vi "Actor Core.vi"(8 "error in":errorcluster, 11 "Zen Analytics in":refnum<class "Zen Analytics.lvclass">) -> (0 "error out":errorcluster, 3 "Actor out":refnum<class "Actor.lvclass">)   [LabVIEW 2019, in "Zen Analytics.lvlib" / "Zen Analytics.lvclass"]
doc: "(<B>Filename</B>: Actor Framework.lvlib:Actor.lvclass:Actor Core.vi)\n\nReceives messages to the actor, reacts to them, and initiates any error handling that may shut the actor down.\n\nDescendant classes may override this VI to append parallel tasks for the actor to complete while it handles messages. Overrides use the Call Parent Method node."
uses:
  Zen Analytics.lvclass
  <vilib>/ActorFramework/Actor/Actor.lvclass
  <vilib>/ActorFramework/Message Enqueuer/Message Enqueuer.lvclass
  Dependency/Plot Cluster.ctl
  Dependency/GraphReff.ctl
  Dependency/Initialize_Cluster.ctl
  Dependency/JSON Cluster(Int).ctl
  Dependency/Shift Registers Cluster.ctl
  <vilib>/ActorFramework/Stop Msg/Stop Msg.lvclass
  Dependency/AnalyticsDataToSM.ctl
  <userlib>/_OpenG.lib/array/array.llb/Empty Array (Variant)__ogtk.vi
  C:/Program Files/National Instruments/LabVIEW 2019/vi.lib/ActorFramework/Actor/Actor.lvclass
panel:
  out "Terminal Count":u32
  out "Reduced 2D":dbl[][](array[numeric])
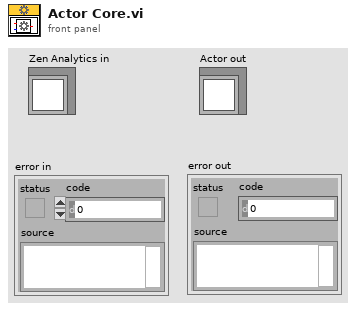
[diagram p1: front panel]
types:
  T1 = cluster{"InitializationParams":cluster{"ColumnNo":i32, "MeasurementData":cluster{"Measurement ID":i32, "Measurement Name":string, "Nominal Values":dbl, "LSL":dbl, "USL":dbl, "LCL":dbl, "UCL":dbl}[]}}
  T2 = enum32{"invalid app kind", "Development System", "Run Time System", "Student Edition", "Embedded LabVIEW", "Evaluation", "Custom"}
  T3 = enum32{"Invalid", "Standard", "Closed", "Hidden", "Minimized", "Maximized"}
  T4 = typedef "Zen Analytics.lvlib/Zen Analytics.lvclass/AnalyticsDataToSM.ctl" = cluster{"Actor Info":cluster{"Analytics Enqueuer":refnum<class "Message Enqueuer.lvclass">, "This VI":refnum<vi>, "Module name":string}, "Statistical Info":string[][], "Graph Refference's":T5, "ErrorMessage":string}
  T5 = typedef "Zen Analytics.lvlib/Zen Analytics.lvclass/GraphReff.ctl" = cluster{"HistgramGraph-reff":refnum<vi>[], "BarGraph-reff":refnum<vi>[], "PieGraph-reff":refnum<vi>[], "Lable-reff":refnum<vi>[], "TrendGraph-reff":refnum<vi>[], "CpCpkTable":refnum<vi>}
  T6 = cluster{"InitializationParams":cluster{"CurrentPartNumber":string, "Re-Initialize?":bool, "MeasurementData":cluster{"Measurement ID":i32, "Measurement Name":string, "Nominal Values":dbl, "LSL":dbl, "USL":dbl, "LCL":dbl, "UCL":dbl}[]}}
  T7 = cluster{"SumOfSquareOfData":dbl, "SumOfMeasurementData":dbl, "N ":u32}
  T8 = typedef "Zen Analytics.lvlib/Zen Analytics.lvclass/Shift Registers Cluster.ctl" = cluster{"Initialize 2D Array":dbl[][], "Analytics Button Pressed?":bool, "Analytics Or Back?":bool, "Read Config":bool, "Prev Terminal Count":u32, "Plot:Present Terminal":u32, "Timeout?":bool, "Re-initialized":bool}
  T9 = typedef "Zen Analytics.lvlib/Zen Analytics.lvclass/JSON Cluster(Int).ctl" = cluster{"Rows In 2D Array":i32, "Columns In 2D Array":i32, "Samples To Display":i32, "Update Rate (Time)":i32, "Update Rate (Samples)":i32, "CurrentPartNumber":string, "AnalyticsDataFormat":cluster{"AnalyticsParameters":cluster{"UpdateRateCategories":cluster{"LOW":cluster{"SampleElapsed":dbl, "TimeElapsed":dbl}, "MEDIUM":cluster{"SampleElapsed":dbl, "TimeElapsed":dbl}, "HIGH":cluster{"SampleElapsed":dbl, "TimeElapsed":dbl}}, "AnalyticsForPartsList":cluster{"Name":string, "InitializationValues":cluster{"RowsIn2DArray":dbl, "ColumnsIn2DArray":dbl, "SamplesToDisplay":dbl, "UpdateRate":string}, "PlotParameters":cluster{"Trend":cluster{"TrendPlotID":dbl, "PlotProperties":cluster{"FontName":string, "FontSize":dbl, "FontColor":string, "IsBold":bool, "IsItalic":bool, "PlotColor":string}}[], "Histogram":cluster{"HistogramPlotID":dbl, "PlotProperties":cluster{"FontName":string, "FontSize":dbl, "FontColor":string, "IsBold":bool, "IsItalic":bool, "PlotColor":string}}[], "BarPlot":cluster{"BarPlotID":dbl, "BarValuesID":dbl, "PlotProperties":cluster{"FontName":string, "FontSize":dbl, "IsBold":bool, "IsItalic":bool, "FontColor":string}, "Sectors":string[]}[], "PieChart":cluster{"PieChartID":dbl, "PieChartValueID":dbl, "PlotProperties":cluster{"FontName":string, "FontSize":dbl, "IsBold":bool, "IsItalic":bool, "FontColor":string}, "Sectors":string[]}[]}}[]}}, "MeasurementData":cluster{"Measurement ID":i32, "Measurement Name":string, "Nominal Values":dbl, "LSL":dbl, "USL":dbl, "LCL":dbl, "UCL":dbl}[], "PlotParameters":cluster{"Trend":cluster{"TrendPlotID":dbl, "PlotProperties":cluster{"FontName":string, "FontSize":dbl, "FontColor":string, "IsBold":bool, "IsItalic":bool, "PlotColor":string}}[], "Histogram":cluster{"HistogramPlotID":dbl, "PlotProperties":cluster{"FontName":string, "FontSize":dbl, "FontColor":string, "IsBold":bool, "IsItalic":bool, "PlotColor":string}}[], "BarPlot":cluster{"BarPlotID":dbl, "BarValuesID":dbl, "PlotProperties":cluster{"FontName":string, "FontSize":dbl, "IsBold":bool, "IsItalic":bool, "FontColor":string}, "Sectors":string[]}[], "PieChart":cluster{"PieChartID":dbl, "PieChartValueID":dbl, "PlotProperties":cluster{"FontName":string, "FontSize":dbl, "IsBold":bool, "IsItalic":bool, "FontColor":string}, "Sectors":string[]}[]}}
  T10 = typedef "Zen Analytics.lvlib/Zen Analytics.lvclass/Initialize_Cluster.ctl" = cluster{"Initialization Values ":cluster{"InitializationParams":cluster{"CurrentPartNumber":string, "Re-Initialize?":bool, "MeasurementData":cluster{"Measurement ID":i32, "Measurement Name":string, "Nominal Values":dbl, "LSL":dbl, "USL":dbl, "LCL":dbl, "UCL":dbl}[]}}}
  T11 = typedef "Zen Analytics.lvlib/Zen Analytics.lvclass/Plot Cluster.ctl" = cluster{"Reduced 2D":dbl[][], "Start Index":i32, "No Of New Termnals":i32, "Top/Bottom":bool, "Values Inserted":i32, "Re-Initialised":bool, "Statistical params":string[][], "MeasurementInitializationData":cluster{"Measurement-ID":i32[], "Measurement Names":string[], "NominalValues":dbl[], "LSL":dbl[], "USL":dbl[], "LCL":dbl[], "UCL":dbl[]}, "MeasurementData":cluster{"Measurement ID":i32, "Measurement Name":string, "Nominal Values":dbl, "LSL":dbl, "USL":dbl, "LCL":dbl, "UCL":dbl}[], "ResultData2D":dbl[][], "PlotParameters":cluster{"Trend":cluster{"TrendPlotID":dbl, "PlotProperties":cluster{"FontName":string, "FontSize":dbl, "FontColor":string, "IsBold":bool, "IsItalic":bool, "PlotColor":string}}[], "Histogram":cluster{"HistogramPlotID":dbl, "PlotProperties":cluster{"FontName":string, "FontSize":dbl, "FontColor":string, "IsBold":bool, "IsItalic":bool, "PlotColor":string}}[], "BarPlot":cluster{"BarPlotID":dbl, "BarValuesID":dbl, "PlotProperties":cluster{"FontName":string, "FontSize":dbl, "IsBold":bool, "IsItalic":bool, "FontColor":string}, "Sectors":string[]}[], "PieChart":cluster{"PieChartID":dbl, "PieChartValueID":dbl, "PlotProperties":cluster{"FontName":string, "FontSize":dbl, "IsBold":bool, "IsItalic":bool, "FontColor":string}, "Sectors":string[]}[]}}
  T12 = cluster{"Core":cluster{"Current VI Reference":refnum<vi>, "Close Panel on Exit?":bool}, "clusterForShiftReg":T8, "JSON Cluster":T9, "Initialization Values":T10, "ResultCluster":cluster{"Terminal Count":u32, "isPass":bool, "Terminal Data 1D":dbl[], "Defect":bool[]}, "Pause Data":bool, "Statistical Parameters":string[][], "InitializationValues":dbl[][], "InitializationValue-PieCahrt":cluster{"InitializationDefect":dbl[], "InitializationProduction":dbl[]}, "InitializationValue-Barplot":cluster{"InitializationDefect":dbl[], "InitializationProduction":dbl[]}, "GraphRefference":T5, "Count":i32, "A_Count":i32, "Data & ID's":cluster{"Measurement-ID":i32[], "Measurement Names":string[], "NominalValues":dbl[], "LSL":dbl[], "USL":dbl[], "LCL":dbl[], "UCL":dbl[]}, "IndexOfMeasurement":i32, "Plot Cluster":T11, "InitializationValues_New":dbl[][], "InterActorData":variant, "StatDataIn ":cluster{"SumOfSquareOfData":dbl, "SumOfMeasurementData":dbl, "N ":u32}[], "StatData Old":cluster{"SumOfSquareOfData":dbl, "SumOfMeasurementData":dbl, "N ":u32}[], "oldTerminalCount":i32}
  T13 = cluster{"SumOfSquareOfData":dbl, "SumOfMeasurementData":dbl, "N ":u32}[]
  T14 = cluster{"Measurement-ID":i32[], "Measurement Names":string[], "NominalValues":dbl[], "LSL":dbl[], "USL":dbl[], "LCL":dbl[], "UCL":dbl[]}
  T15 = cluster{"InitializationDefect":dbl[], "InitializationProduction":dbl[]}
  T16 = cluster{"Terminal Count":u32, "isPass":bool, "Terminal Data 1D":dbl[], "Defect":bool[]}
  T17 = cluster{"Current VI Reference":refnum<vi>, "Close Panel on Exit?":bool}
  T18 = cluster{"AnalyticsParameters":cluster{"UpdateRateCategories":cluster{"LOW":cluster{"SampleElapsed":dbl, "TimeElapsed":dbl}, "MEDIUM":cluster{"SampleElapsed":dbl, "TimeElapsed":dbl}, "HIGH":cluster{"SampleElapsed":dbl, "TimeElapsed":dbl}}, "AnalyticsForPartsList":cluster{"Name":string, "InitializationValues":cluster{"RowsIn2DArray":dbl, "ColumnsIn2DArray":dbl, "SamplesToDisplay":dbl, "UpdateRate":string}, "PlotParameters":cluster{"Trend":cluster{"TrendPlotID":dbl, "PlotProperties":cluster{"FontName":string, "FontSize":dbl, "FontColor":string, "IsBold":bool, "IsItalic":bool, "PlotColor":string}}[], "Histogram":cluster{"HistogramPlotID":dbl, "PlotProperties":cluster{"FontName":string, "FontSize":dbl, "FontColor":string, "IsBold":bool, "IsItalic":bool, "PlotColor":string}}[], "BarPlot":cluster{"BarPlotID":dbl, "BarValuesID":dbl, "PlotProperties":cluster{"FontName":string, "FontSize":dbl, "IsBold":bool, "IsItalic":bool, "FontColor":string}, "Sectors":string[]}[], "PieChart":cluster{"PieChartID":dbl, "PieChartValueID":dbl, "PlotProperties":cluster{"FontName":string, "FontSize":dbl, "IsBold":bool, "IsItalic":bool, "FontColor":string}, "Sectors":string[]}[]}}[]}}
  T19 = cluster{"Trend":cluster{"TrendPlotID":dbl, "PlotProperties":cluster{"FontName":string, "FontSize":dbl, "FontColor":string, "IsBold":bool, "IsItalic":bool, "PlotColor":string}}[], "Histogram":cluster{"HistogramPlotID":dbl, "PlotProperties":cluster{"FontName":string, "FontSize":dbl, "FontColor":string, "IsBold":bool, "IsItalic":bool, "PlotColor":string}}[], "BarPlot":cluster{"BarPlotID":dbl, "BarValuesID":dbl, "PlotProperties":cluster{"FontName":string, "FontSize":dbl, "IsBold":bool, "IsItalic":bool, "FontColor":string}, "Sectors":string[]}[], "PieChart":cluster{"PieChartID":dbl, "PieChartValueID":dbl, "PlotProperties":cluster{"FontName":string, "FontSize":dbl, "IsBold":bool, "IsItalic":bool, "FontColor":string}, "Sectors":string[]}[]}
  T20 = cluster{"Measurement ID":i32, "Measurement Name":string, "Nominal Values":dbl, "LSL":dbl, "USL":dbl, "LCL":dbl, "UCL":dbl}[]
  T21 = typedef "Zen Analytics.lvlib/Zen Analytics.lvclass/Json Partno Specific output.ctl" = cluster{"Array Params ":cluster{"RowsIn2DArray":i32, "ColumnsIn2DArray":i32, "SamplesToDisplay":i32, "UpdateRate":string}, "PlotParameters":cluster{"Trend":cluster{"TrendPlotID":dbl, "PlotProperties":cluster{"FontName":string, "FontSize":dbl, "FontColor":string, "IsBold":bool, "IsItalic":bool, "PlotColor":string}}[], "Histogram":cluster{"HistogramPlotID":dbl, "PlotProperties":cluster{"FontName":string, "FontSize":dbl, "FontColor":string, "IsBold":bool, "IsItalic":bool, "PlotColor":string}}[], "BarPlot":cluster{"BarPlotID":dbl, "BarValuesID":dbl, "PlotProperties":cluster{"FontName":string, "FontSize":dbl, "IsBold":bool, "IsItalic":bool, "FontColor":string}, "Sectors":string[]}[], "PieChart":cluster{"PieChartID":dbl, "PieChartValueID":dbl, "PlotProperties":cluster{"FontName":string, "FontSize":dbl, "IsBold":bool, "IsItalic":bool, "FontColor":string}, "Sectors":string[]}[]}}
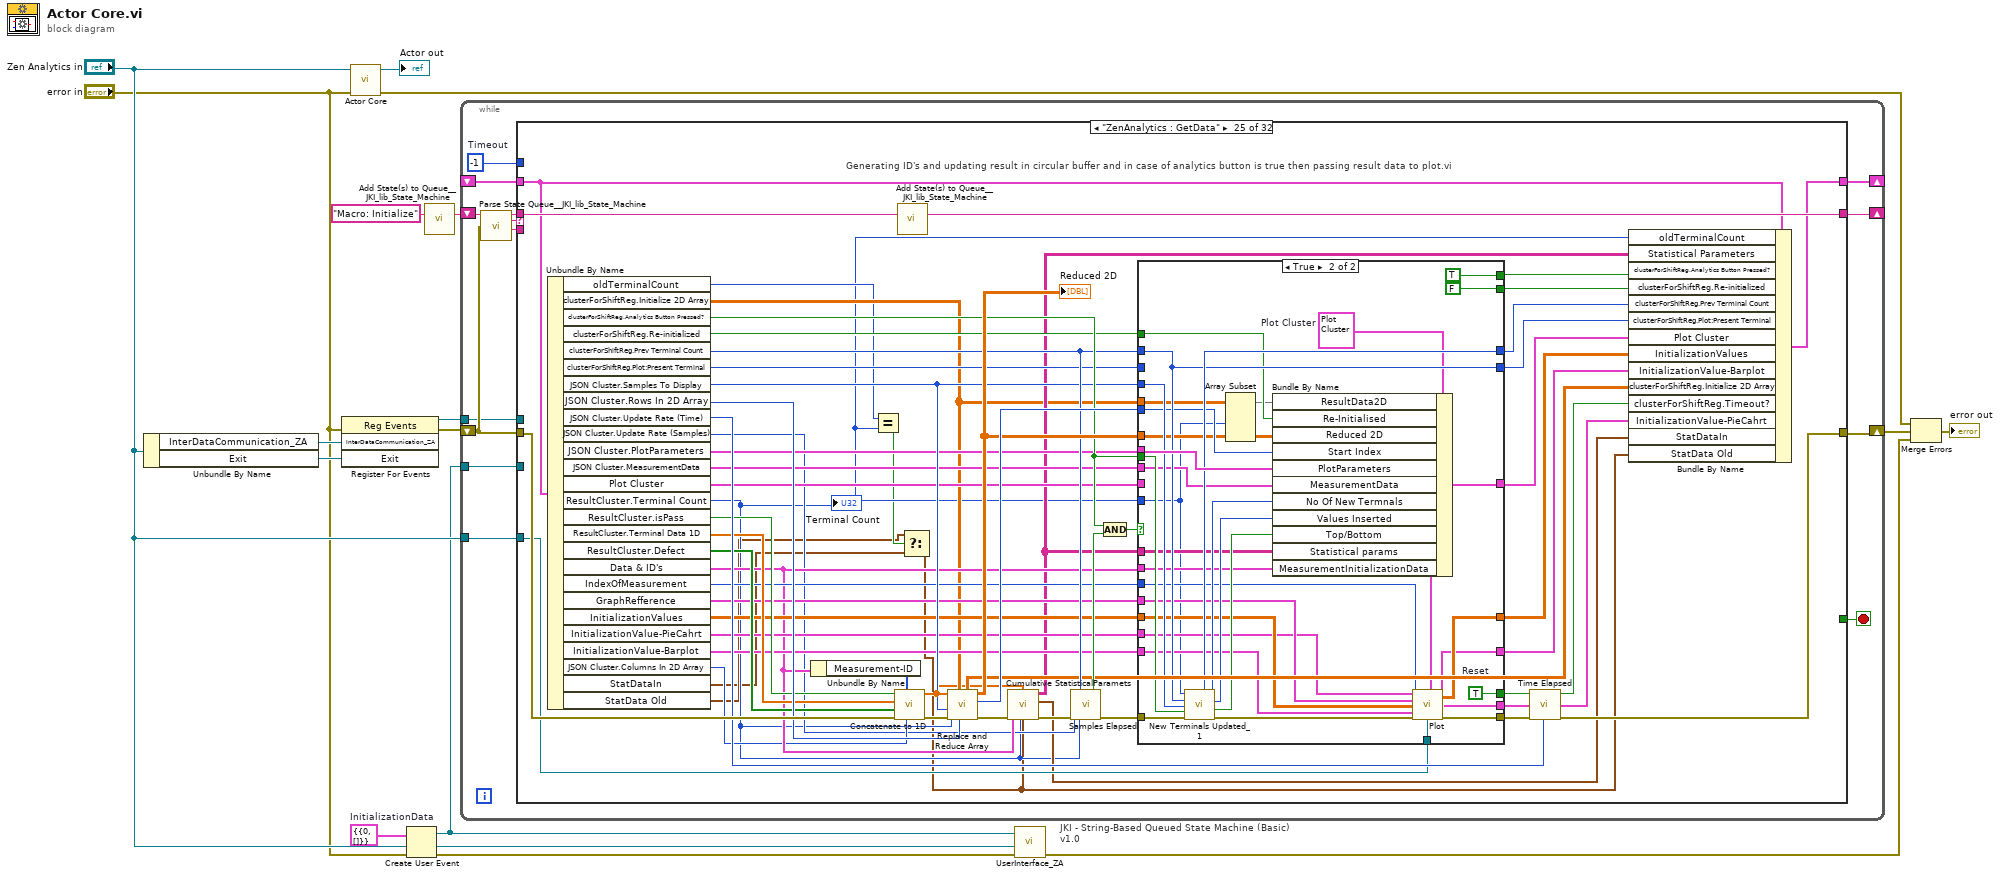
[diagram p0: block diagram]
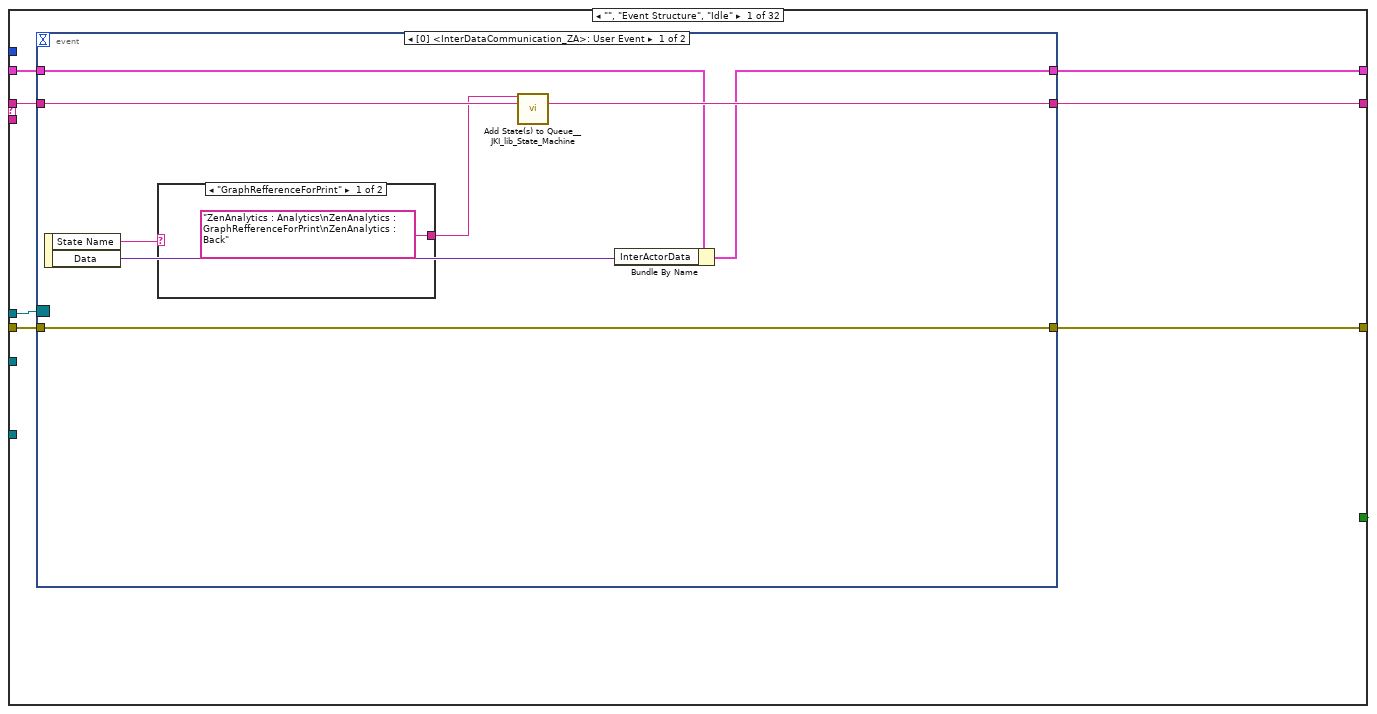
[diagram p2: hidden frame]
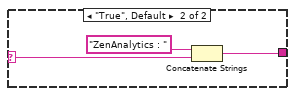
[diagram p3: hidden frame]
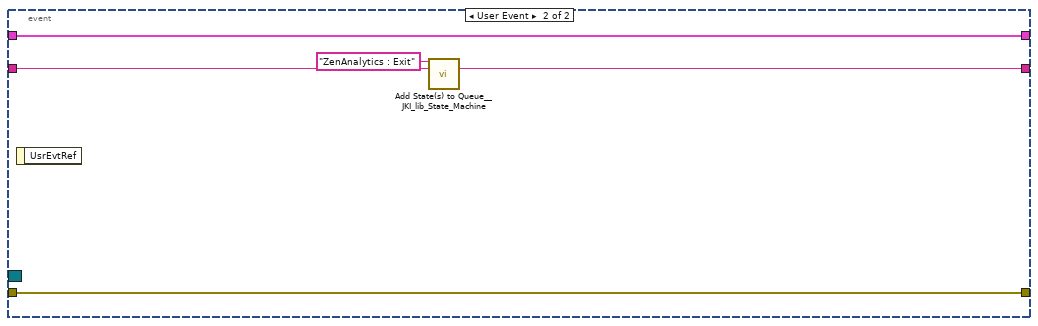
[diagram p4: hidden frame]
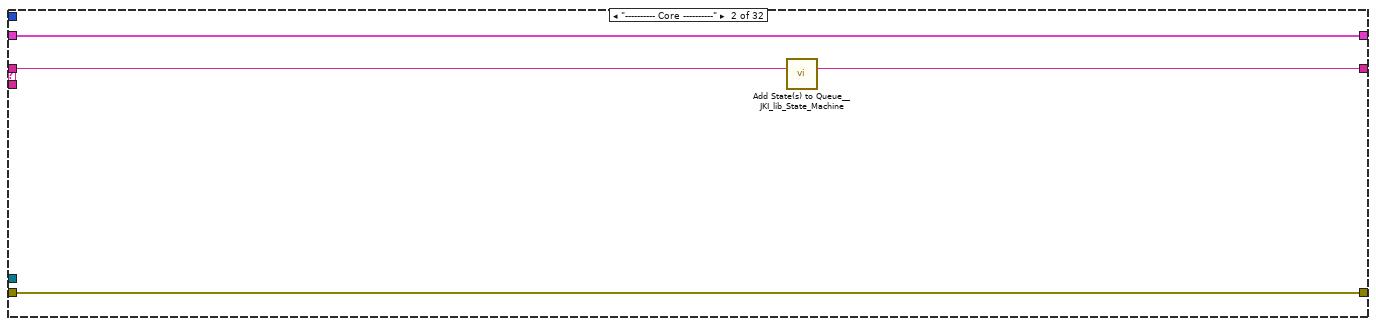
[diagram p5: hidden frame]
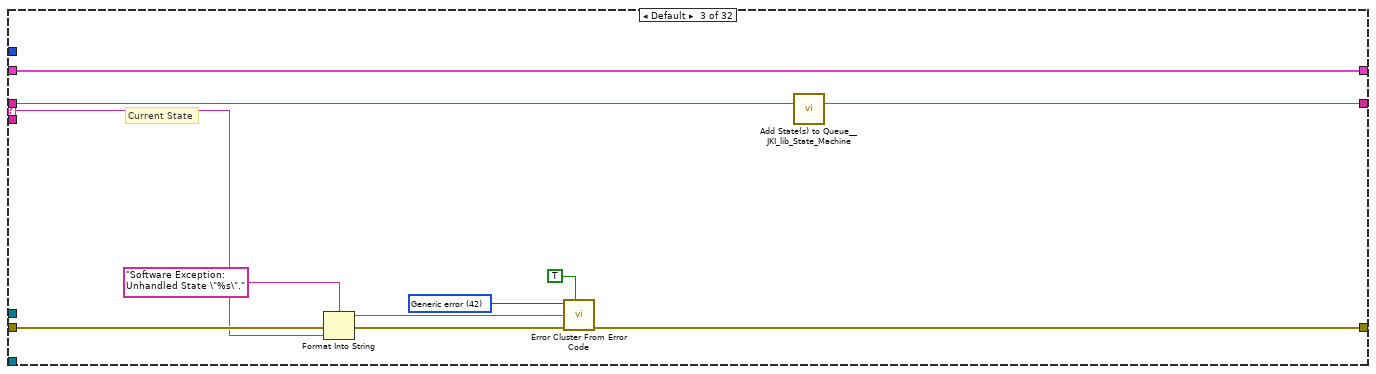
[diagram p6: hidden frame]
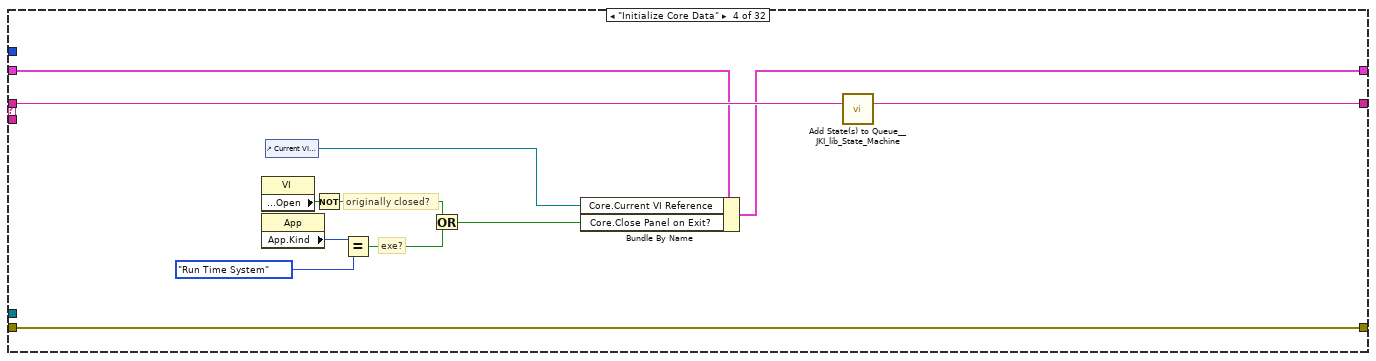
[diagram p7: hidden frame]
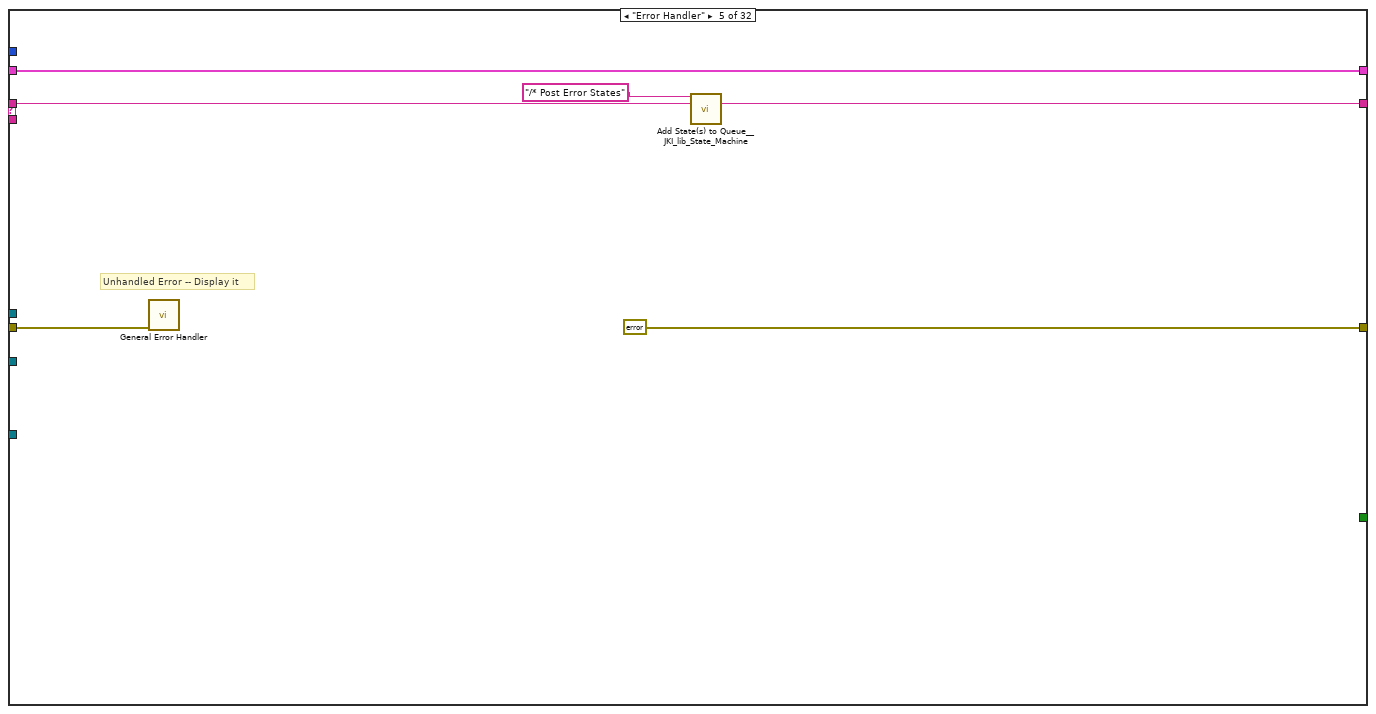
[diagram p8: hidden frame]
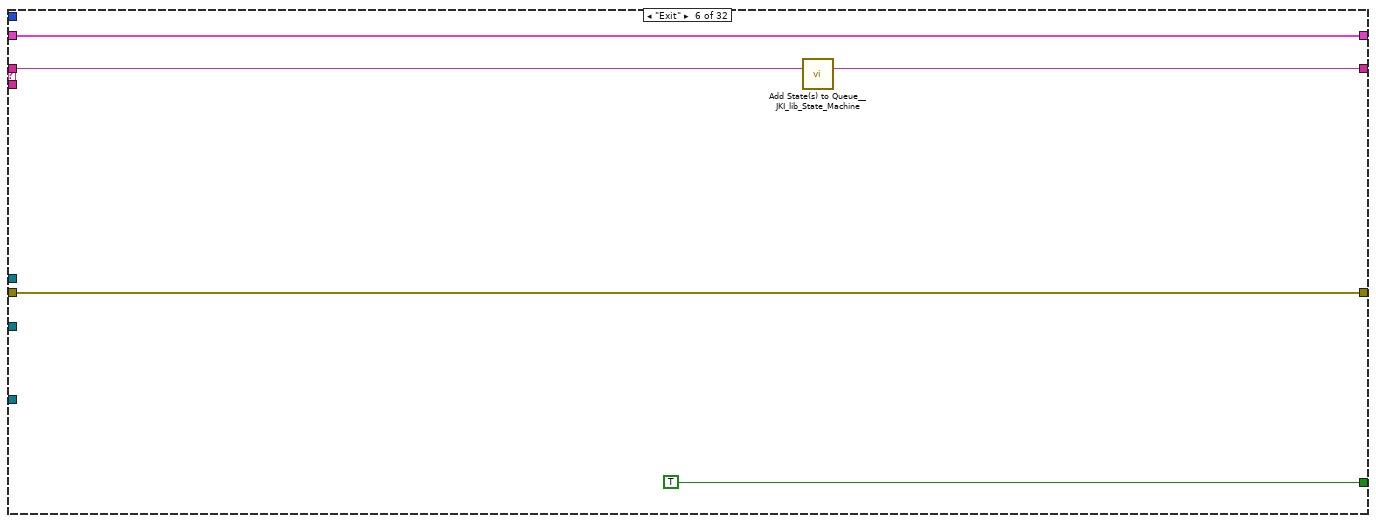
[diagram p9: hidden frame]
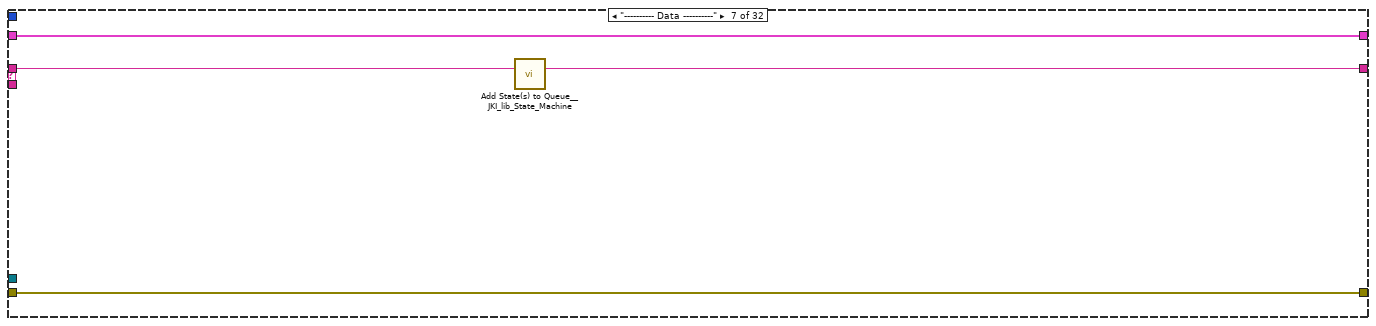
[diagram p10: hidden frame]
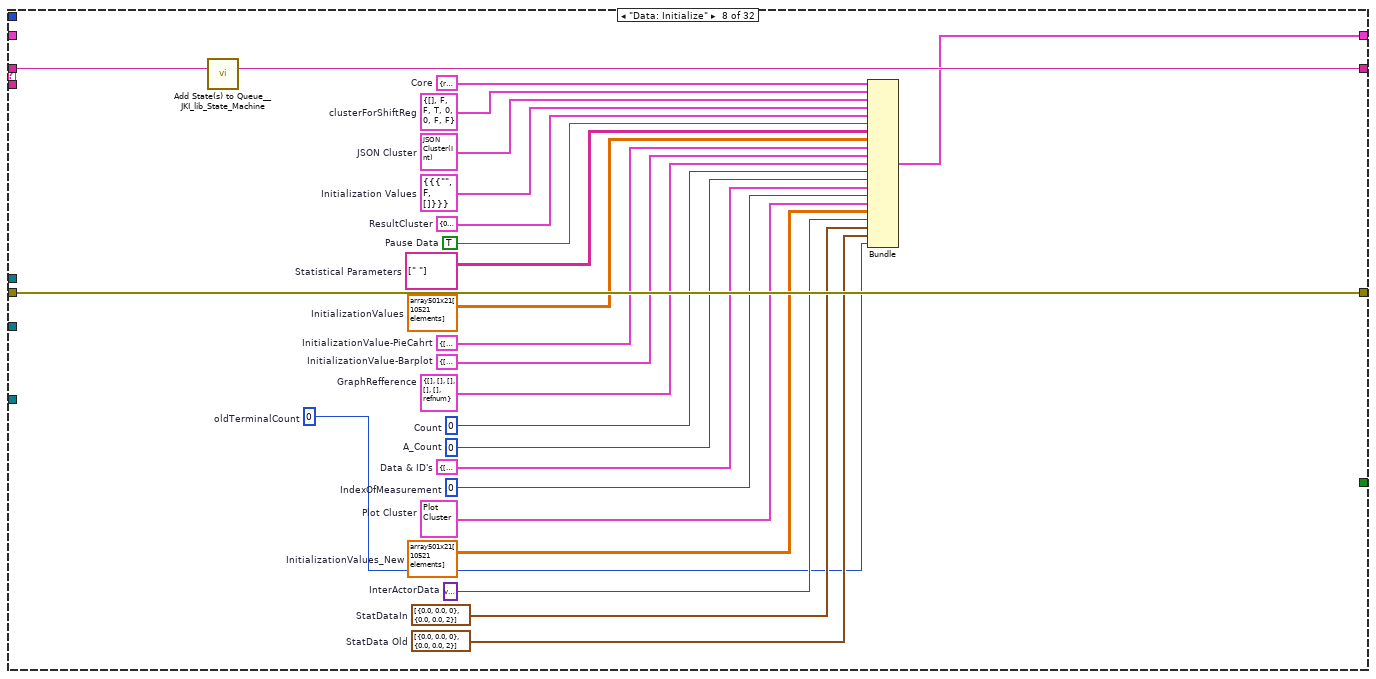
[diagram p11: hidden frame]
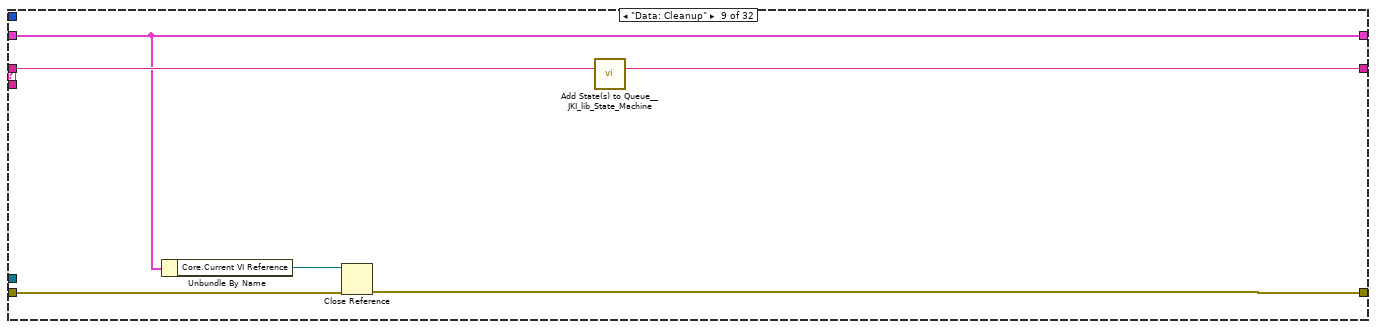
[diagram p12: hidden frame]
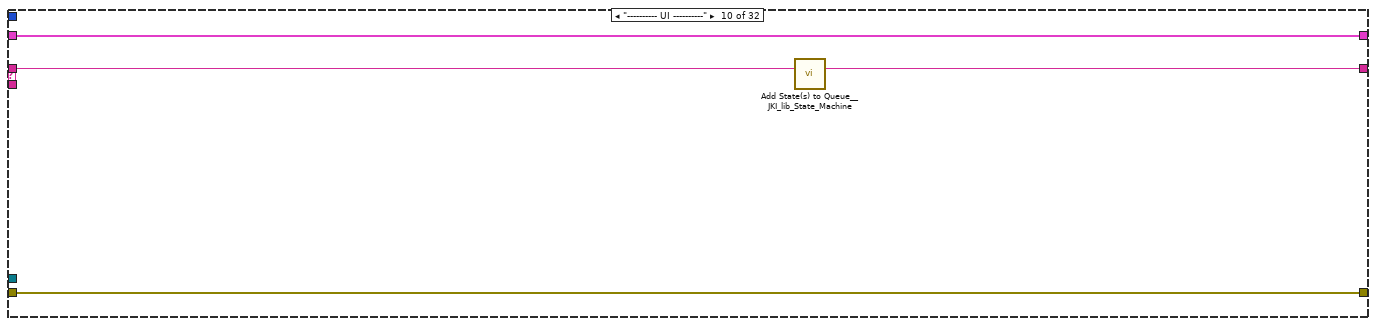
[diagram p13: hidden frame]
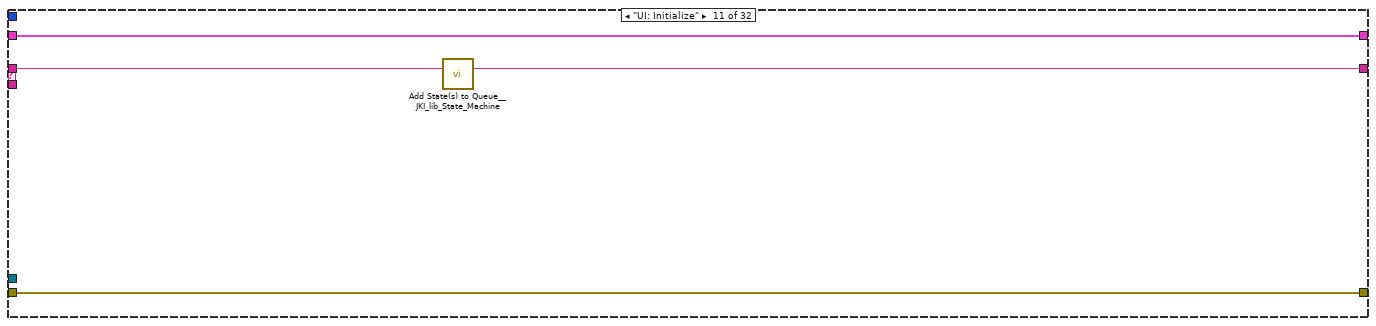
[diagram p14: hidden frame]
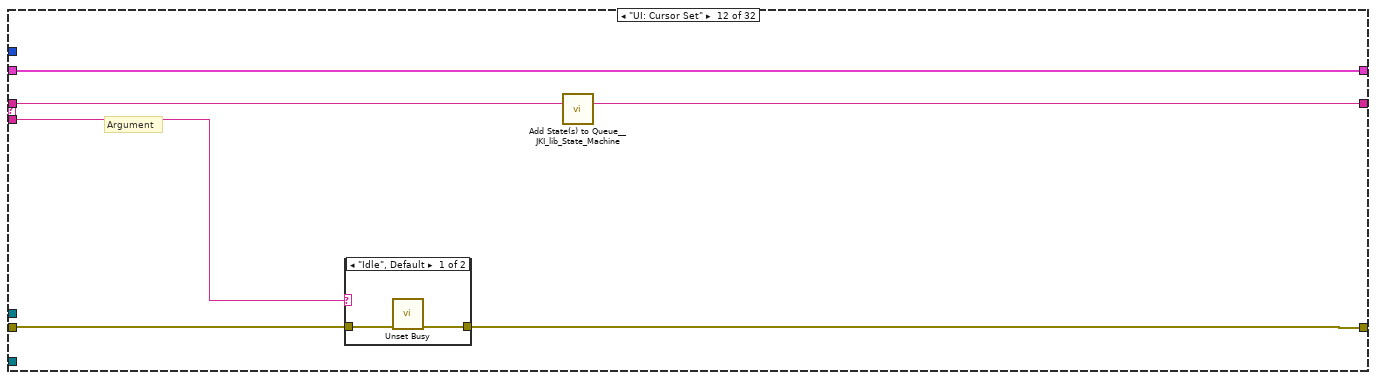
[diagram p15: hidden frame]
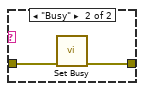
[diagram p16: hidden frame]
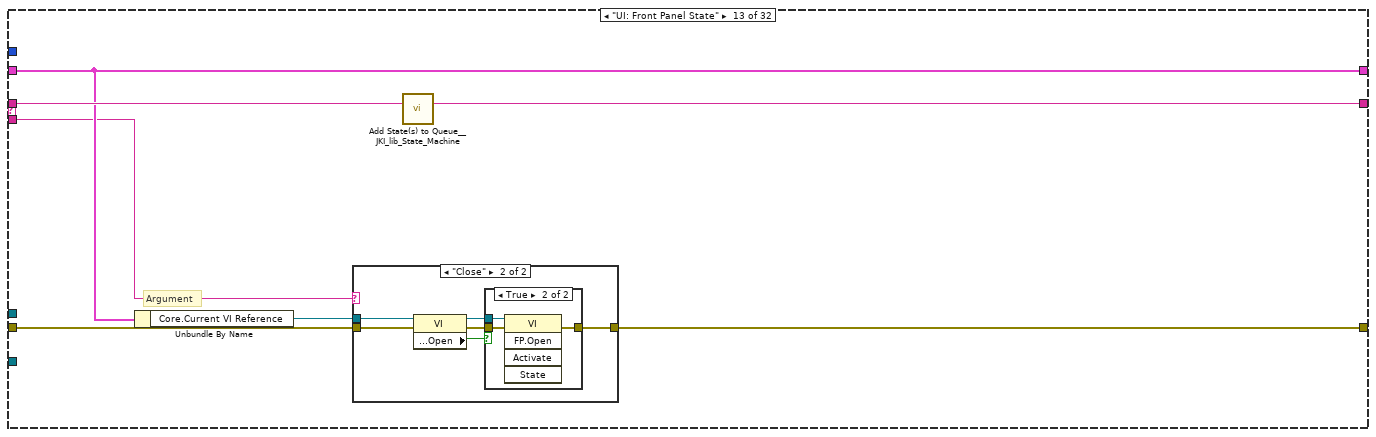
[diagram p17: hidden frame]
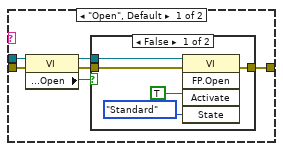
[diagram p18: hidden frame]
diagram:
  w6 = T1 {"InitializationParams"={"ColumnNo"=0, "MeasurementData"=[]}}  # InitializationData
  n1 = Unbundle By Name("Zen Analytics in") -> ("InterDataCommunication_ZA"=w9:refnum<user-event>, "Exit"=w7:refnum<user-event>)
  n2 = register-events(error in="error in", w9, w7) -> (reference out=w13:refnum<event-registration>, error out=w5:errorcluster)  [unwired: 1 in]
  n3 = call-parent "Actor Core.vi"("error in"="error in", "Actor in"="Zen Analytics in") -> ("error out"=w12:errorcluster, "Actor out"=→"Actor out":refnum<class "Actor.lvclass">)  [unwired: 8 in]
  n4 = Create User Event(user event datatype=w6, error in="error in") -> (user event=w2:refnum<user-event>, error out=w4:errorcluster)
  n5 = call <vilib>:"Add State(s) to Queue__JKI_lib_State_Machine.vi"("State(s) in (\"\")"="Macro: Initialize") -> ("States Out"=w15:string)  [unwired: 14 in]
  n6 = while "JKI - String-Based Queued State Machine (Basic) v1.0" {
    shift-right: [w23] -> _
    shift-left: _ -> [w22]
    shift-right: [w26] -> w1
    shift-left: w5 -> [w19]
    shift-right: [w25] -> _
    shift-left: w15 -> [w27]
    tunnel: "Zen Analytics in" -> [w20]
    tunnel: w13 -> [w18]
    tunnel: w2 -> [w17]
    stop <- w24 stop-if-true
    w21 = -1  # Timeout
    n7 = call <vilib>:"Parse State Queue__JKI_lib_State_Machine.vi"("State Queue"=w27, "Error In (no error)"=w19) -> ("Remaining States"=w29:string, "Current State"=w30:string, "Arguments"=w28:string)  [unwired: 11 in]
    n8 = case shown="\"ZenAnalytics : GetData\"" w30 {
      selector: w30 -> [_ _ w60 _ _ _ _ _ _ _ _ _ _ _ _ _ _ _ _ _ _ _ _ _ _ _ _ _ _ _ _ _]
      tunnel: w29 -> [w34 w59 w64 w82 w88 w93 w97 w122 w128 w132 w136 w142 w153 w179 w184 w194 w198 w231 w252 w262 w310 w401 w417 w427 w487 w547 w553 w568 w586 w597 w610 w620]
      tunnel: w28 -> [_ _ _ _ _ _ _ _ _ _ _ w137 w147 _ _ _ _ _ _ _ _ _ _ _ _ _ _ _ _ _ _ _]
      tunnel: w22 -> [w35 w56 w62 w73 w85 w91 w94 _ w123 w129 w134 w140 w149 w176 w181 w191 w195 w229 w251 w258 w294 w397 w413 w423 w472 w536 w551 w565 w578 w589 w602 w619]
      tunnel: [w36 w57 w66 w79 errorcluster {"status"=FALSE, "code"=0, "source"=""} ("error out") w90 w95 w119 w124 w130 w133 w138 w150 w177 w182 w192 w196 w211 w243 w254 w280 w399 w415 w425 w480 w542 w550 w563 w583 w598 w599 w612] -> w26
      tunnel: w19 -> [w37 w57 w65 w79 w84 w90 w95 w119 w125 w130 w133 w139 w151 w177 w182 w192 w196 w228 w244 w261 w282 w400 w416 w426 w474 w542 w550 w558 w577 w598 w599 w613]
      tunnel: [w32 w58 w63 w81 w87 w92 w96 w121 w127 w131 w135 w141 w152 w178 w183 w193 w197 w232 w253 w263 w309 w402 w418 w428 w486 w546 w552 w567 w585 w596 w609 w621] -> w25
      tunnel: [FALSE _ _ _ _ TRUE _ _ _ _ _ _ _ _ _ _ _ _ _ _ _ _ _ _ _ _ _ _ _ _ _ _] -> w24
      tunnel: [w33 w56 w62 w80 w85 w91 w94 w120 w123 w129 w134 w140 w149 w176 w181 w191 w195 w230 w251 w257 w283 w396 w412 w422 w483 w535 w551 w564 w578 w588 w601 w619] -> w23
      tunnel: w21 -> [_ _ _ _ _ _ _ _ _ _ _ _ _ _ _ _ _ _ _ _ _ _ _ _ _ _ _ _ _ _ _ _]
      tunnel: w20 -> [_ _ _ _ _ _ _ _ _ _ _ _ _ _ _ _ _ w208 w246 _ w273 w392 _ _ w439 _ _ w566 w584 _ _ w618]
      tunnel: w18 -> [w38 _ _ _ _ _ _ _ _ _ _ _ _ _ _ _ _ _ _ _ _ _ _ _ _ _ _ _ _ _ _ w614]
      tunnel: w17 -> [_ _ _ _ _ _ _ _ _ _ _ _ _ _ _ _ _ _ _ _ w275 _ _ _ _ _ _ _ _ _ _ _]
      frame "", "Event Structure", "Idle" {
        n9 = event shown="[0] <InterDataCommunication_ZA>: User Event" {
          selector: w38 -> [_ _]
          dyn-events: _ -> [_ _]
          timeout: _ -> [_ _]
          tunnel: [w42 w51] -> w36
          tunnel: w37 -> [w42 w51]
          tunnel: w35 -> [w43 w55]
          tunnel: w34 -> [w45 w53]
          tunnel: [w44 w55] -> w33
          tunnel: [w46 w52] -> w32
          event User Event {
            n10 = event-data() -> ("State Name"=w39:string, "Data"=w41:variant)  [unwired: 1 in]
            n11 = case shown="\"GraphRefferenceForPrint\"" w39 {
              selector: w39 -> [_ w48]
              tunnel: ["ZenAnalytics : Analytics\nZenAnalytics : GraphRefferenceForPrint\nZenAnalytics : Back" w49] -> w40
              frame "GraphRefferenceForPrint" {
              }
              frame "True", Default {
                n12 = Concatenate Strings("ZenAnalytics : " ("State(s) in Front (\"\")"), w48) -> (w49:string)
              }
            }
            n13 = call <vilib>:"Add State(s) to Queue__JKI_lib_State_Machine.vi"("State(s) in Front (\"\")"=w40, "State(s) in (\"\")"=w45) -> ("States Out"=w46:string)  [unwired: 13 in]
            n14 = Bundle By Name(cluster=w43, "InterActorData"=w41) -> (w44:T12)
          }
          event User Event {
            n15 = event-data() -> ()  [unwired: 1 in, 1 out]
            n16 = call <vilib>:"Add State(s) to Queue__JKI_lib_State_Machine.vi"("State(s) in Front (\"\")"="ZenAnalytics : Exit" ("State(s) in Front (\"\")"), "State(s) in (\"\")"=w53) -> ("States Out"=w52:string)  [unwired: 13 in]
          }
        }
      }
      frame "---------- Core ----------" {
        n17 = call <vilib>:"Add State(s) to Queue__JKI_lib_State_Machine.vi"("State(s) in (\"\")"=w59) -> ("States Out"=w58:string)  [unwired: 14 in]
      }
      frame Default {
        w69 = 42 items=["No error", "Argument error", "Memory is full", "Out of zone", "End of file", "File already open", "Generic file I/O error", "File not found", "File permission error", "Disk is full", "Duplicate path", "Too many files open", "System feature not enabled", "Resource file not found", "Cannot add resource", "Resource not found", "Image not found", "Image memory error", "Pen does not exist", "Config type invalid", "Config token not found", "Config parse error", "Config memory error", "Bad external code format", "Bad external code offset", "External code not present", "Null window", "Destroy window error", "Null menu", "Print aborted", "Bad print record", "Print driver error", "Windows error during printing", "Memory error during printing", "Print dialog error", "Generic print error", "Invalid device refnum", "Device not found", "Device parameter error", "Device unit error", "Cannot open device", "Device call aborted", "Generic error", "Cancelled by user", "Object ID too low", "Object ID too high", "Object not in heap", "Unknown heap", "Unknown object (invalid DefProc)", "Unknown object (DefProc not in table)", "Message out of range", "Invalid (null) method", "Unknown message", "Manager call not supported", "Bad address", "Network operation in progress", "Network operation timed out", "Connection is busy", "Network attribute not supported", "Network error", "Address in use", "System out of memory", "Connection aborted", "Connection refused", "Not connected", "Already connected", "Connection closed", "Initialization error (interapplication manager)", "Bad occurrence", "Wait on unbound occurrence handler", "Occurrence queue overflow", "Datalog type conflict", "Unused", "Unrecognized type (interapplication manager)", "Memory corrupt", "Failed to make temporary DLL", "Old CIN version", "Drag socket not found", "Failed to load drop-object", "Failed to register OLE object", "Failed to release OLE object", "Format specifier type mismatch", "Unknown format specifier", "Too few format specifiers", "Too many format specifiers", "Scan failed", "Newer CIN version", "Error converting to variant", "Runtime menu error", "Password tampered", "Variant attribute not found", "Incompatible variant data type", "Event data is not available", "Event Store is not present", "Occurrence is not found", "Event Queue is not created", "Event info is not available", "Refnum passed is NULL", "Error retrieving Class GUID", "Error retrieving CoClass GUID", "Error retrieving TypeLib GUID.", "Bad built application magic bytes.", "Specific driver is different from the specific driver associated with the Logical Name.", "There is no session opened to the class driver.", "Max Error", "MAX - Error with config objects", "MAX - Error loading configuration", "MAX - Group not supported"]
        # "Current State"
        n18 = Format Into String(format string="Software Exception: Unhandled State \"%s\"." ("message"), error in=w65, w60) -> (resulting string=w68:string, error out=w67:errorcluster)  [unwired: 1 in]
        n19 = call <vilib>:"Error Cluster From Error Code.vi"("show call chain? (False)"=TRUE, "error in (no error)"=w67, "error message (\"\")"=w68, "error code (0)"=w69) -> ("error out"=w66:errorcluster)  [unwired: 5 in]
        n20 = call <vilib>:"Add State(s) to Queue__JKI_lib_State_Machine.vi"("State(s) in (\"\")"=w64) -> ("States Out"=w63:string)  [unwired: 14 in]
      }
      frame "Initialize Core Data" {
        # "originally closed?"
        # "exe?"
        n21 = property class="VI"() -> ("Front Panel.Open"=w78:bool)  [unwired: 2 in, 2 out]
        n22 = property class="App"() -> ("App.Kind"=w77:T2)  [unwired: 2 in, 2 out]
        n23 = control-ref of="Current VI Reference"() -> (w71:refnum<vi>)
        n24 = Not(x=w78) -> (.not. x?=w75:bool)
        n25 = Equal?(x=w77, y=T2."Run Time System" ("Application:Kind")) -> (x = y?=w74:bool)
        n26 = Or(x=w75, y=w74) -> (x .or. y?=w72:bool)
        n27 = Bundle By Name(cluster=w73, "Core.Current VI Reference"=w71, "Core.Close Panel on Exit?"=w72) -> (w80:T12)
        n28 = call <vilib>:"Add State(s) to Queue__JKI_lib_State_Machine.vi"("State(s) in (\"\")"=w82) -> ("States Out"=w81:string)  [unwired: 14 in]
      }
      frame "Error Handler" {
        # "Unhandled Error -- Display it"
        # "Clear error"
        n29 = call <vilib>:"General Error Handler.vi"("error in (no error)"=w84) -> ()  [unwired: 10 in, 5 out]
        n30 = call <vilib>:"Add State(s) to Queue__JKI_lib_State_Machine.vi"("State(s) in Front (\"\")"="/* Post Error States", "State(s) in (\"\")"=w88) -> ("States Out"=w87:string)  [unwired: 13 in]
      }
      frame "Exit" {
        n31 = call <vilib>:"Add State(s) to Queue__JKI_lib_State_Machine.vi"("State(s) in (\"\")"=w93) -> ("States Out"=w92:string)  [unwired: 14 in]
      }
      frame "---------- Data ----------" {
        n32 = call <vilib>:"Add State(s) to Queue__JKI_lib_State_Machine.vi"("State(s) in (\"\")"=w97) -> ("States Out"=w96:string)  [unwired: 14 in]
      }
      frame "Data: Initialize" {
        w98 = 0  # oldTerminalCount
        w99 = T13 [{"SumOfSquareOfData"=0.0, "SumOfMeasurementData"=0.0, "N "=0}, {"SumOfSquareOfData"=0.0, "SumOfMeasurementData"=0.0, "N "=2}]  # StatData Old
        w100 = T13 [{"SumOfSquareOfData"=0.0, "SumOfMeasurementData"=0.0, "N "=0}, {"SumOfSquareOfData"=0.0, "SumOfMeasurementData"=0.0, "N "=2}]  # StatDataIn
        w101 = variant  # InterActorData
        w102 = dbl[][] array501x21[10521 elements]  # InitializationValues_New
        w103 = T11 {"Reduced 2D"=[], "Start Index"=0, "No Of New Termnals"=0, "Top/Bottom"=FALSE, "Values Inserted"=0, "Re-Initialised"=FALSE, "Statistical params"=[], "MeasurementInitializationData"={"Measurement-ID"=[], "Measurement Names"=[], "NominalValues"=[], "LSL"=[], "USL"=[], "LCL"=[], "UCL"=[]}, "MeasurementData"=[], "ResultData2D"=[], "PlotParameters"={"Trend"=[], "Histogram"=[], "BarPlot"=[], "PieChart"=[]}}  # Plot Cluster
        w104 = T5 {"HistgramGraph-reff"=[], "BarGraph-reff"=[], "PieGraph-reff"=[], "Lable-reff"=[], "TrendGraph-reff"=[], "CpCpkTable"=refnum}  # GraphRefference
        w105 = 0  # IndexOfMeasurement
        w106 = T14 {"Measurement-ID"=[], "Measurement Names"=[], "NominalValues"=[], "LSL"=[], "USL"=[], "LCL"=[], "UCL"=[]}  # Data & ID's
        w107 = 0  # A_Count
        w108 = 0  # Count
        w109 = T15 {"InitializationDefect"=[0.0, 0.0, 0.0, 0.0, 0.0, 0.0, 0.0, 0.0, 0.0, 0.0, 0.0, 0.0, 0.0, 0.0, 0.0, 0.0, 0.0, 0.0, 0.0, 0.0, 0.0, 0.0, 0.0, 0.0, 0.0, 0.0, 0.0, 0.0, 0.0, 0.0, 0.0, 0.0, 0.0, 0.0, 0.0, 0.0, 0.0, 0.0, 0.0, 0.0, 0.0, 0.0, 0.0, 0.0, 0.0, 0.0, 0.0, 0.0, 0.0, 0.0, 0.0, 0.0, 0.0, 0.0, 0.0, 0.0, 0.0, 0.0, 0.0, 0.0, 0.0, 0.0, 0.0, 0.0, 0.0, 0.0, 0.0, 0.0, 0.0, 0.0, 0.0, 0.0, 0.0, 0.0, 0.0, 0.0, 0.0, 0.0, 0.0, 0.0, 0.0, 0.0, 0.0, 0.0, 0.0, 0.0, 0.0, 0.0, 0.0, 0.0, 0.0, 0.0, 0.0, 0.0, 0.0, 0.0, 0.0, 0.0, 0.0, 0.0, 0.0, 0.0, 0.0, 0.0, 0.0, 0.0, 0.0, 0.0, 0.0, 0.0, 0.0, 0.0, 0.0, 0.0, 0.0, 0.0, 0.0, 0.0, 0.0, 0.0, 0.0, 0.0, 0.0, 0.0, 0.0, 0.0, 0.0, 0.0, 0.0, 0.0, 0.0, 0.0, 0.0, 0.0, 0.0, 0.0, 0.0, 0.0, 0.0, 0.0, 0.0, 0.0, 0.0, 0.0, 0.0, 0.0, 0.0, 0.0, 0.0, 0.0, 0.0, 0.0, 0.0, 0.0, 0.0, 0.0, 0.0, 0.0, 0.0, 0.0, 0.0, 0.0, 0.0, 0.0, 0.0, 0.0, 0.0, 0.0, 0.0, 0.0, 0.0, 0.0, 0.0, 0.0, 0.0, 0.0, 0.0, 0.0, 0.0, 0.0, 0.0, 0.0, 0.0, 0.0, 0.0, 0.0, 0.0, 0.0, 0.0, 0.0, 0.0, 0.0, 0.0, 0.0, 0.0, 0.0, 0.0, 0.0, 0.0, 0.0, 0.0, 0.0, 0.0, 0.0, 0.0, 0.0, 0.0, 0.0, 0.0, 0.0, 0.0, 0.0, 0.0, 0.0, 0.0, 0.0, 0.0, 0.0, 0.0, 0.0, 0.0, 0.0, 0.0, 0.0, 0.0, 0.0, 0.0, 0.0, 0.0, 0.0, 0.0, 0.0, 0.0, 0.0, 0.0, 0.0, 0.0, 0.0, 0.0, 0.0, 0.0, 0.0, 0.0, 0.0, 0.0, 0.0, 0.0, 0.0, 0.0, 0.0, 0.0, 0.0, 0.0, 0.0, 0.0, 0.0, 0.0, 0.0, 0.0, 0.0, 0.0, 0.0, 0.0, 0.0, 0.0, 0.0, 0.0, 0.0, 0.0, 0.0, 0.0, 0.0, 0.0, 0.0, 0.0, 0.0, 0.0, 0.0, 0.0, 0.0, 0.0, 0.0, 0.0, 0.0, 0.0, 0.0, 0.0, 0.0, 0.0, 0.0, 0.0, 0.0, 0.0, 0.0, 0.0, 0.0, 0.0, 0.0, 0.0, 0.0, 0.0, 0.0, 0.0, 0.0, 0.0, 0.0, 0.0, 0.0, 0.0, 0.0, 0.0, 0.0, 0.0, 0.0, 0.0, 0.0, 0.0, 0.0, 0.0, 0.0, 0.0, 0.0, 0.0, 0.0, 0.0, 0.0, 0.0, 0.0, 0.0, 0.0, 0.0, 0.0, 0.0, 0.0, 0.0, 0.0, 0.0, 0.0, 0.0, 0.0, 0.0, 0.0, 0.0, 0.0, 0.0, 0.0, 0.0, 0.0, 0.0, 0.0, 0.0, 0.0, 0.0, 0.0, 0.0, 0.0, 0.0, 0.0, 0.0, 0.0, 0.0, 0.0, 0.0, 0.0, 0.0, 0.0, 0.0, 0.0, 0.0, 0.0, 0.0, 0.0, 0.0, 0.0, 0.0, 0.0, 0.0, 0.0, 0.0, 0.0, 0.0, 0.0, 0.0, 0.0, 0.0, 0.0, 0.0, 0.0, 0.0, 0.0, 0.0, 0.0, 0.0, 0.0, 0.0, 0.0, 0.0, 0.0, 0.0, 0.0, 0.0, 0.0, 0.0, 0.0, 0.0, 0.0, 0.0, 0.0, 0.0, 0.0, 0.0, 0.0, 0.0, 0.0, 0.0, 0.0, 0.0, 0.0, 0.0, 0.0, 0.0, 0.0, 0.0, 0.0, 0.0, 0.0, 0.0, 0.0, 0.0, 0.0, 0.0, 0.0, 0.0, 0.0, 0.0, 0.0, 0.0, 0.0, 0.0, 0.0, 0.0, 0.0, 0.0, 0.0, 0.0, 0.0, 0.0, 0.0, 0.0, 0.0, 0.0, 0.0, 0.0, 0.0, 0.0, 0.0, 0.0, 0.0, 0.0, 0.0, 0.0, 0.0, 0.0, 0.0, 0.0, 0.0, 0.0, 0.0, 0.0, 0.0, 0.0, 0.0, 0.0, 0.0, 0.0, 0.0, 0.0, 0.0, 0.0, 0.0, 0.0, 0.0, 0.0, 0.0, 0.0, 0.0, 0.0, 0.0, 0.0, 0.0, 0.0, 0.0, 0.0, 0.0, 0.0, 0.0, 0.0, 0.0, 0.0, 0.0, 0.0], "InitializationProduction"=[0.0, 0.0, 0.0, 0.0, 0.0, 0.0, 0.0, 0.0, 0.0, 0.0, 0.0, 0.0, 0.0, 0.0, 0.0, 0.0, 0.0, 0.0, 0.0, 0.0, 0.0]}  # InitializationValue-Barplot
        w110 = T15 {"InitializationDefect"=[0.0, 0.0, 0.0, 0.0, 0.0, 0.0, 0.0, 0.0, 0.0, 0.0, 0.0, 0.0, 0.0, 0.0, 0.0, 0.0, 0.0, 0.0, 0.0, 0.0, 0.0, 0.0, 0.0, 0.0, 0.0, 0.0, 0.0, 0.0, 0.0, 0.0, 0.0, 0.0, 0.0, 0.0, 0.0, 0.0, 0.0, 0.0, 0.0, 0.0, 0.0, 0.0, 0.0, 0.0, 0.0, 0.0, 0.0, 0.0, 0.0, 0.0, 0.0, 0.0, 0.0, 0.0, 0.0, 0.0, 0.0, 0.0, 0.0, 0.0, 0.0, 0.0, 0.0, 0.0, 0.0, 0.0, 0.0, 0.0, 0.0, 0.0, 0.0, 0.0, 0.0, 0.0, 0.0, 0.0, 0.0, 0.0, 0.0, 0.0, 0.0, 0.0, 0.0, 0.0, 0.0, 0.0, 0.0, 0.0, 0.0, 0.0, 0.0, 0.0, 0.0, 0.0, 0.0, 0.0, 0.0, 0.0, 0.0, 0.0, 0.0, 0.0, 0.0, 0.0, 0.0, 0.0, 0.0, 0.0, 0.0, 0.0, 0.0, 0.0, 0.0, 0.0, 0.0, 0.0, 0.0, 0.0, 0.0, 0.0, 0.0, 0.0, 0.0, 0.0, 0.0, 0.0, 0.0, 0.0, 0.0, 0.0, 0.0, 0.0, 0.0, 0.0, 0.0, 0.0, 0.0, 0.0, 0.0, 0.0, 0.0, 0.0, 0.0, 0.0, 0.0, 0.0, 0.0, 0.0, 0.0, 0.0, 0.0, 0.0, 0.0, 0.0, 0.0, 0.0, 0.0, 0.0, 0.0, 0.0, 0.0, 0.0, 0.0, 0.0, 0.0, 0.0, 0.0, 0.0, 0.0, 0.0, 0.0, 0.0, 0.0, 0.0, 0.0, 0.0, 0.0, 0.0, 0.0, 0.0, 0.0, 0.0, 0.0, 0.0, 0.0, 0.0, 0.0, 0.0, 0.0, 0.0, 0.0, 0.0, 0.0, 0.0, 0.0, 0.0, 0.0, 0.0, 0.0, 0.0, 0.0, 0.0, 0.0, 0.0, 0.0, 0.0, 0.0, 0.0, 0.0, 0.0, 0.0, 0.0, 0.0, 0.0, 0.0, 0.0, 0.0, 0.0, 0.0, 0.0, 0.0, 0.0, 0.0, 0.0, 0.0, 0.0, 0.0, 0.0, 0.0, 0.0, 0.0, 0.0, 0.0, 0.0, 0.0, 0.0, 0.0, 0.0, 0.0, 0.0, 0.0, 0.0, 0.0, 0.0, 0.0, 0.0, 0.0, 0.0, 0.0, 0.0, 0.0, 0.0, 0.0, 0.0, 0.0, 0.0, 0.0, 0.0, 0.0, 0.0, 0.0, 0.0, 0.0, 0.0, 0.0, 0.0, 0.0, 0.0, 0.0, 0.0, 0.0, 0.0, 0.0, 0.0, 0.0, 0.0, 0.0, 0.0, 0.0, 0.0, 0.0, 0.0, 0.0, 0.0, 0.0, 0.0, 0.0, 0.0, 0.0, 0.0, 0.0, 0.0, 0.0, 0.0, 0.0, 0.0, 0.0, 0.0, 0.0, 0.0, 0.0, 0.0, 0.0, 0.0, 0.0, 0.0, 0.0, 0.0, 0.0, 0.0, 0.0, 0.0, 0.0, 0.0, 0.0, 0.0, 0.0, 0.0, 0.0, 0.0, 0.0, 0.0, 0.0, 0.0, 0.0, 0.0, 0.0, 0.0, 0.0, 0.0, 0.0, 0.0, 0.0, 0.0, 0.0, 0.0, 0.0, 0.0, 0.0, 0.0, 0.0, 0.0, 0.0, 0.0, 0.0, 0.0, 0.0, 0.0, 0.0, 0.0, 0.0, 0.0, 0.0, 0.0, 0.0, 0.0, 0.0, 0.0, 0.0, 0.0, 0.0, 0.0, 0.0, 0.0, 0.0, 0.0, 0.0, 0.0, 0.0, 0.0, 0.0, 0.0, 0.0, 0.0, 0.0, 0.0, 0.0, 0.0, 0.0, 0.0, 0.0, 0.0, 0.0, 0.0, 0.0, 0.0, 0.0, 0.0, 0.0, 0.0, 0.0, 0.0, 0.0, 0.0, 0.0, 0.0, 0.0, 0.0, 0.0, 0.0, 0.0, 0.0, 0.0, 0.0, 0.0, 0.0, 0.0, 0.0, 0.0, 0.0, 0.0, 0.0, 0.0, 0.0, 0.0, 0.0, 0.0, 0.0, 0.0, 0.0, 0.0, 0.0, 0.0, 0.0, 0.0, 0.0, 0.0, 0.0, 0.0, 0.0, 0.0, 0.0, 0.0, 0.0, 0.0, 0.0, 0.0, 0.0, 0.0, 0.0, 0.0, 0.0, 0.0, 0.0, 0.0, 0.0, 0.0, 0.0, 0.0, 0.0, 0.0, 0.0, 0.0, 0.0, 0.0, 0.0, 0.0, 0.0, 0.0, 0.0, 0.0, 0.0, 0.0, 0.0, 0.0, 0.0, 0.0, 0.0, 0.0, 0.0, 0.0, 0.0, 0.0, 0.0, 0.0, 0.0, 0.0, 0.0, 0.0, 0.0, 0.0, 0.0, 0.0, 0.0, 0.0, 0.0, 0.0, 0.0, 0.0, 0.0, 0.0, 0.0, 0.0, 0.0, 0.0, 0.0, 0.0, 0.0, 0.0, 0.0, 0.0], "InitializationProduction"=[0.0, 0.0, 0.0, 0.0, 0.0, 0.0, 0.0, 0.0, 0.0, 0.0, 0.0, 0.0, 0.0, 0.0, 0.0, 0.0, 0.0, 0.0, 0.0, 0.0, 0.0]}  # InitializationValue-PieCahrt
        w111 = dbl[][] array501x21[10521 elements]  # InitializationValues
        w112 = string[][] [[" "]]  # Statistical Parameters
        w113 = TRUE  # Pause Data
        w114 = T16 {"Terminal Count"=0, "isPass"=FALSE, "Terminal Data 1D"=[], "Defect"=[]}  # ResultCluster
        w115 = T10 {"Initialization Values "={"InitializationParams"={"CurrentPartNumber"="", "Re-Initialize?"=FALSE, "MeasurementData"=[]}}}  # Initialization Values
        w116 = T9 {"Rows In 2D Array"=0, "Columns In 2D Array"=0, "Samples To Display"=0, "Update Rate (Time)"=0, "Update Rate (Samples)"=0, "CurrentPartNumber"="", "AnalyticsDataFormat"={"AnalyticsParameters"={"UpdateRateCategories"={"LOW"={"SampleElapsed"=0.0, "TimeElapsed"=0.0}, "MEDIUM"={"SampleElapsed"=0.0, "TimeElapsed"=0.0}, "HIGH"={"SampleElapsed"=0.0, "TimeElapsed"=0.0}}, "AnalyticsForPartsList"=[]}}, "MeasurementData"=[], "PlotParameters"={"Trend"=[], "Histogram"=[], "BarPlot"=[], "PieChart"=[]}}  # JSON Cluster
        w117 = T8 {"Initialize 2D Array"=[], "Analytics Button Pressed?"=FALSE, "Analytics Or Back?"=FALSE, "Read Config"=TRUE, "Prev Terminal Count"=0, "Plot:Present Terminal"=0, "Timeout?"=FALSE, "Re-initialized"=FALSE}  # clusterForShiftReg
        w118 = T17 {"Current VI Reference"=refnum, "Close Panel on Exit?"=FALSE}  # Core
        n33 = call <vilib>:"Add State(s) to Queue__JKI_lib_State_Machine.vi"("State(s) in (\"\")"=w122) -> ("States Out"=w121:string)  [unwired: 14 in]
        n34 = Bundle("Core"=w118, "clusterForShiftReg"=w117, "JSON Cluster"=w116, "Initialization Values"=w115, "ResultCluster"=w114, "Pause Data"=w113, "Statistical Parameters"=w112, "InitializationValues"=w111, "InitializationValue-PieCahrt"=w110, "InitializationValue-Barplot"=w109, "GraphRefference"=w104, "Count"=w108, "A_Count"=w107, "Data & ID's"=w106, "IndexOfMeasurement"=w105, "Plot Cluster"=w103, "InitializationValues_New"=w102, "InterActorData"=w101, "StatDataIn"=w100, "StatData Old"=w99, "oldTerminalCount"=w98) -> (w120:T12)  [unwired: 1 in]
      }
      frame "Data: Cleanup" {
        n35 = Unbundle By Name(w123) -> ("Core.Current VI Reference"=w126:refnum<vi>)
        n36 = Close Reference(reference=w126, error in (no error)=w125) -> (error out=w124:errorcluster)
        n37 = call <vilib>:"Add State(s) to Queue__JKI_lib_State_Machine.vi"("State(s) in (\"\")"=w128) -> ("States Out"=w127:string)  [unwired: 14 in]
      }
      frame "---------- UI ----------" {
        n38 = call <vilib>:"Add State(s) to Queue__JKI_lib_State_Machine.vi"("State(s) in (\"\")"=w132) -> ("States Out"=w131:string)  [unwired: 14 in]
      }
      frame "UI: Initialize" {
        n39 = call <vilib>:"Add State(s) to Queue__JKI_lib_State_Machine.vi"("State(s) in (\"\")"=w136) -> ("States Out"=w135:string)  [unwired: 14 in]
      }
      frame "UI: Cursor Set" {
        # "Argument"
        n40 = case shown="\"Idle\", Default" w137 {
          tunnel: w139 -> [w144 w146]
          tunnel: [w143 w145] -> w138
          frame "Idle", Default {
            n41 = call <vilib>:"Unset Busy.vi"("error in (no error)"=w144) -> ("error out"=w143:errorcluster)  [unwired: 10 in]
          }
          frame "Busy" {
            n42 = call <vilib>:"Set Busy.vi"("error in (no error)"=w146) -> ("error out"=w145:errorcluster)  [unwired: 9 in, 1 out]
          }
        }
        n43 = call <vilib>:"Add State(s) to Queue__JKI_lib_State_Machine.vi"("State(s) in (\"\")"=w142) -> ("States Out"=w141:string)  [unwired: 14 in]
      }
      frame "UI: Front Panel State" {
        # "Argument"
        n44 = Unbundle By Name(w149) -> ("Core.Current VI Reference"=w148:refnum<vi>)
        n45 = case shown="\"Close\"" w147 {
          tunnel: w151 -> [w157 w170]
          tunnel: [w159 w171] -> w150
          tunnel: w148 -> [w158 w168]
          frame "Open", Default {
            n46 = property class="VI"(reference=w158, error in=w157) -> (reference out=w155:refnum<vi>, error out=w156:errorcluster, "Front Panel.Open"=w154:bool)
            n47 = case shown="False" w154 {
              tunnel: [w162 w165] -> w159
              tunnel: w156 -> [w161 w165]
              tunnel: w155 -> [w160 _]
              frame False {
                n48 = invoke class="VI" method="FP.Open"(reference=w160, error in=w161, "Activate"=TRUE, "State"=T3."Standard") -> (error out=w162:errorcluster)  [unwired: 1 in, 4 out]
              }
              frame True {
              }
            }
          }
          frame "Close" {
            n49 = property class="VI"(reference=w168, error in=w170) -> (reference out=w167:refnum<vi>, error out=w169:errorcluster, "Front Panel.Open"=w166:bool)
            n50 = case shown="True" w166 {
              tunnel: [w172 w175] -> w171
              tunnel: w169 -> [w172 w174]
              tunnel: w167 -> [_ w173]
              frame False {
              }
              frame True {
                n51 = invoke class="VI" method="FP.Open"(reference=w173, error in=w174) -> (error out=w175:errorcluster)  [unwired: 3 in, 4 out]
              }
            }
          }
        }
        n52 = call <vilib>:"Add State(s) to Queue__JKI_lib_State_Machine.vi"("State(s) in (\"\")"=w153) -> ("States Out"=w152:string)  [unwired: 14 in]
      }
      frame "---------- Macro ----------" {
        n53 = call <vilib>:"Add State(s) to Queue__JKI_lib_State_Machine.vi"("State(s) in (\"\")"=w179) -> ("States Out"=w178:string)  [unwired: 14 in]
      }
      frame "Macro: Initialize" {
        w180 = "Data: Initialize\nInitialize Core Data\nUI: Initialize\nUI: Front Panel State >> Close\nZenAnalytics : JSONRead\nZenAnalytics : ActorInfo"  # Data: Initialize Initialize Core Data UI: Initialize UI: Front Panel State >> Close ZenAnalytics : JSONRead ZenAnalytics : ActorInfo
        n54 = call <vilib>:"Add State(s) to Queue__JKI_lib_State_Machine.vi"("State(s) in Front (\"\")"=w180, "State(s) in (\"\")"=w184) -> ("States Out"=w183:string)  [unwired: 13 in]
      }
      frame "Macro: Exit" {
        n55 = Unbundle By Name(w191) -> ("Core.Close Panel on Exit?"=w190:bool)
        n56 = Select(t="UI: Front Panel State >> Close", s=w190, f="") -> (s? t:f=w187:string)
        n57 = call <vilib>:"Add State(s) to Queue__JKI_lib_State_Machine.vi"("State(s) in (\"\")"=w187, "State(s) at Back (\"\")"="Data: Cleanup\nExit") -> ("States Out"=w185:string)  [unwired: 13 in]
        n58 = call <vilib>:"Add State(s) to Queue__JKI_lib_State_Machine.vi"("State(s) in Front (\"\")"=w185, "State(s) in (\"\")"=w194) -> ("States Out"=w193:string)  [unwired: 13 in]
      }
      frame "---------- ZenAnalytics----------" {
        n59 = call <vilib>:"Add State(s) to Queue__JKI_lib_State_Machine.vi"("State(s) in (\"\")"=w198) -> ("States Out"=w197:string)  [unwired: 14 in]
      }
      frame "ZenAnalytics : JSONRead" {
        # "Read JSON file"
        n60 = call <vilib>:"Application Directory.vi"() -> ("Application Directory"=w224:path)
        n61 = Build Path(base path=w224, name or relative path="Configuration file\\Analytics Parameters.json") -> (appended path=w199:path)
        n62 = Concatenate Strings("Check JSON file path/File name !" ("SolutionForError"), "\r", "ErrorCode:", "0X0E00A100" ("ErrorCode")) -> (w214:string)
        n63 = call <vilib>:"File to Variant.vi"("JSON FilePath"=w199, "error in (no error)"=w228) -> ("JSON Variant"=w225:variant, "error out"=w213:errorcluster)  [unwired: 6 in, 1 out]
        n64 = Bundle By Name(cluster=T4 {"Actor Info"={"Analytics Enqueuer"=refnum, "This VI"=refnum, "Module name"=""}, "Statistical Info"=[], "Graph Refference's"={"HistgramGraph-reff"=[], "BarGraph-reff"=[], "PieGraph-reff"=[], "Lable-reff"=[], "TrendGraph-reff"=[], "CpCpkTable"=refnum}, "ErrorMessage"=""} ("Analytics Information"), "ErrorMessage"=w214) -> (w219:T4)
        n65 = Unbundle By Name(w229) -> ("JSON Cluster.AnalyticsDataFormat"=w227:T18)
        n66 = Unbundle By Name(w213) -> ("status"=w222:bool)
        n67 = case shown="True" w222 {
          tunnel: "ERROR_INFO" ("State") -> [_ w238]
          tunnel: w208 -> [_ w237]
          tunnel: w219 -> [_ w236]
          frame False {
          }
          frame True {
            n68 = call "Output_ZA.vi"("State"=w238, "Analytics Information"=w236, "Zen Analytics in"=w237) -> ()  [unwired: 7 in, 2 out]
          }
        }
        n69 = call <vilib>:"Clear Errors.vi"("error in (no error)"=w213) -> ("error out"=w212:errorcluster)  [unwired: 5 in, 1 out]
        n70 = Variant To Data(error in=w212, type=w227, Variant=w225) -> (data=w226:T18, error out=w210:errorcluster)
        n71 = call <vilib>:"Add State(s) to Queue__JKI_lib_State_Machine.vi"("State(s) in (\"\")"=w231) -> ("States Out"=w232:string)  [unwired: 14 in]
        n72 = Bundle By Name(cluster=w229, "JSON Cluster.AnalyticsDataFormat"=w226) -> (w230:T12)
        n73 = Concatenate Strings("Check JSON Structure and JOSN data type !" ("SolutionForError"), "\r", "ErrorCode:", "0X0E00A101" ("ErrorCode")) -> (w200:string)
        n74 = Bundle By Name(cluster=T4 {"Actor Info"={"Analytics Enqueuer"=refnum, "This VI"=refnum, "Module name"=""}, "Statistical Info"=[], "Graph Refference's"={"HistgramGraph-reff"=[], "BarGraph-reff"=[], "PieGraph-reff"=[], "Lable-reff"=[], "TrendGraph-reff"=[], "CpCpkTable"=refnum}, "ErrorMessage"=""} ("Analytics Information"), "ErrorMessage"=w200) -> (w205:T4)
        n75 = Unbundle By Name(w210) -> ("status"=w209:bool)
        n76 = call <vilib>:"Clear Errors.vi"("error in (no error)"=w210) -> ("error out"=w211:errorcluster)  [unwired: 5 in, 1 out]
        n77 = case shown="True" w209 {
          tunnel: "ERROR_INFO" ("State") -> [_ w235]
          tunnel: w208 -> [_ w234]
          tunnel: w205 -> [_ w233]
          frame False {
          }
          frame True {
            n78 = call "Output_ZA.vi"("State"=w235, "Analytics Information"=w233, "Zen Analytics in"=w234) -> ()  [unwired: 7 in, 2 out]
          }
        }
      }
      frame "ZenAnalytics : ActorInfo" {
        # "Sending Actor info to parent actor"
        n79 = call <vilib>:"Read Self Enqueuer.vi"("Actor"=w246) -> ("Self Enqueuer"=w247:refnum<class "Message Enqueuer.lvclass">)  [unwired: 10 in]
        n80 = call <vilib>:"Application Directory.vi"() -> ("Application Directory"=w242:path)
        n81 = Build Path(base path=w242, name or relative path=path "ZenAnalytics/Zen Analytics/Methods/UserInterface_ZA.vi" ("Path")) -> (appended path=w239:path)
        n82 = Open VI Reference(vi path=w239, error in (no error)=w244) -> (vi reference=w250:refnum<vi>, error out=w245:errorcluster)  [unwired: 4 in]
        n83 = Bundle By Name(cluster=T4 {"Actor Info"={"Analytics Enqueuer"=refnum, "This VI"=refnum, "Module name"=""}, "Statistical Info"=[], "Graph Refference's"={"HistgramGraph-reff"=[], "BarGraph-reff"=[], "PieGraph-reff"=[], "Lable-reff"=[], "TrendGraph-reff"=[], "CpCpkTable"=refnum}, "ErrorMessage"=""} ("Analytics Information"), "Actor Info.Analytics Enqueuer"=w247, "Actor Info.This VI"=w250) -> (w248:T4)
        n84 = call <vilib>:"Add State(s) to Queue__JKI_lib_State_Machine.vi"("State(s) in (\"\")"=w252) -> ("States Out"=w253:string)  [unwired: 14 in]
        n85 = call "Output_ZA.vi"("error in (no error)"=w245, "State"="ACTOR_INFO", "Analytics Information"=w248, "Zen Analytics in"=w246) -> ("error out"=w243:errorcluster)  [unwired: 6 in, 1 out]
      }
      frame "ZenAnalytics : Init" {
        # "Getting the selected part initialization data"
        n86 = Unbundle By Name(w258) -> ("InterActorData"=w260:variant)
        n87 = Variant To Data(error in=w261, type=T6 {"InitializationParams"={"CurrentPartNumber"="", "Re-Initialize?"=FALSE, "MeasurementData"=[]}} ("Initialization Values"), Variant=w260) -> (data=w255:T6, error out=w254:errorcluster)
        n88 = Bundle By Name(cluster=w258, "Initialization Values.Initialization Values"=w255) -> (w257:T12)
        n89 = call <vilib>:"Add State(s) to Queue__JKI_lib_State_Machine.vi"("State(s) in Front (\"\")"="ZenAnalytics : Initialization" ("State(s) in Front (\"\")"), "State(s) in (\"\")"=w262) -> ("States Out"=w263:string)  [unwired: 13 in]
      }
      frame "ZenAnalytics : Initialization" {
        w279 = T1 {"InitializationParams"={"ColumnNo"=0, "MeasurementData"=[]}}  # InitializationData
        # "Initialization of circular buffer and other parameters"
        n90 = Unbundle By Name(w294) -> ("InitializationValue-PieCahrt"=w267:T15, "InitializationValue-Barplot"=w268:T15, "clusterForShiftReg.Re-initialized"=w316:bool, "clusterForShiftReg.Plot:Present Terminal"=w315:u32, "clusterForShiftReg.Prev Terminal Count"=w271:u32, "clusterForShiftReg.Initialize 2D Array"=w314:dbl[][], "clusterForShiftReg.Timeout?"=w311:bool, "clusterForShiftReg.Analytics Button Pressed?"=w312:bool, "clusterForShiftReg.Analytics Or Back?"=w313:bool, "JSON Cluster.Rows In 2D Array"=w307:i32, "JSON Cluster.Samples To Display"=w306:i32, "JSON Cluster.Columns In 2D Array"=w305:i32, "JSON Cluster.Update Rate (Samples)"=w304:i32, "JSON Cluster.Update Rate (Time)"=w303:i32, "JSON Cluster.PlotParameters"=w302:T19, "JSON Cluster.CurrentPartNumber"=w301:string, "Initialization Values.Initialization Values.InitializationParams.Re-Initialize?"=w300:bool, "Initialization Values.Initialization Values.InitializationParams.MeasurementData"=w296:T20, "Initialization Values.Initialization Values.InitializationParams.CurrentPartNumber"=w299:string, "JSON Cluster"=w298:T9, "InitializationValue-Barplot.InitializationDefect"=w297:dbl[], "Data & ID's"=w266:T14, "StatDataIn"=w265:T13)
        n91 = case shown="False" w300 {
          tunnel: [w350 w369] -> w295
          tunnel: w282 -> [w351 w376]
          tunnel: [w341 w383] -> w278
          tunnel: w296 -> [w341 w383]
          tunnel: [w336 w380] -> w293
          tunnel: [w344 w368] -> w292
          tunnel: [w335 w360] -> w277
          tunnel: [w342 w367] -> w289
          tunnel: w302 -> [_ _]
          tunnel: w307 -> [_ _]
          tunnel: w306 -> [_ _]
          tunnel: w305 -> [_ _]
          tunnel: w304 -> [_ _]
          tunnel: w303 -> [_ _]
          tunnel: [w354 w374] -> w291
          tunnel: [w353 w373] -> w290
          tunnel: w299 -> [_ w378]
          tunnel: [w337 w379] -> w274
          tunnel: w314 -> [w338 _]
          tunnel: w301 -> [w352 _]
          tunnel: [w352 w378] -> w288
          tunnel: w298 -> [w348 w371]
          tunnel: w273 -> [_ w366]
          tunnel: [w347 0] -> w272
          tunnel: w271 -> [w347 _]
          tunnel: [w345 w364] -> w270
          tunnel: [w346 w363] -> w269
          tunnel: w268 -> [w346 _]
          tunnel: w267 -> [w345 _]
          tunnel: w266 -> [w333 _]
          tunnel: [w331 w357] -> w264
          tunnel: w265 -> [w332 _]
          frame False {
            n92 = call "Json_Specific part.vi"("error in (no error)"=w351, "JSON Cluster"=w348, "Part-num"=w352) -> ("error out"=w340:errorcluster, "Json Part no specicific op"=w343:T21)  [unwired: 7 in]
            n93 = Unbundle By Name(w343) -> ("Array Params.RowsIn2DArray"=w336:i32, "Array Params.SamplesToDisplay"=w344:i32, "Array Params.ColumnsIn2DArray"=w335:i32, "PlotParameters"=w342:T19)
            n94 = Unbundle By Name(w343) -> ("Array Params.UpdateRate"=w356:string)
            n95 = call "AnalyticsParamCluster.vi"("error in (no error)"=w340, "Number of columns"=w335, "MeasurementData"=w341) -> ("error out"=w339:errorcluster, "Initialization Data"=w334:T14)  [unwired: 6 in, 1 out]
            n96 = call "String To Enum.vi"("error in (no error)"=w340, "string"=w356) -> ("error out"=w355:errorcluster, "Select Update Rate"=w349:enum16{"HIGH", "MEDIUM", "LOW"})  [unwired: 8 in]
            n97 = call "DeleteAndAdd.vi"("Input"=w338, "Old Initialization Data"=w333, "New Initialization Data"=w334, "ColumnSize"=w335, "RowSize"=w336, "error in (no error)"=w339, "StatDataIn"=w332) -> ("StatDataOut"=w331:T13, "Output 2 After Adding"=w337:dbl[][])  [unwired: 10 in, 1 out]
            n98 = call "Rate to Sampls&Time.vi"("error in (no error)"=w355, "JSON Cluster"=w348, "Select Update Rate"=w349) -> ("error out"=w350:errorcluster, "TimeElapsed"=w353:i32, "SampleElapsed"=w354:i32)  [unwired: 6 in]
          }
          frame True {
            w364 = T15 {"InitializationDefect"=[0.0, 0.0, 0.0, 0.0, 0.0, 0.0, 0.0, 0.0, 0.0, 0.0, 0.0, 0.0, 0.0, 0.0, 0.0, 0.0, 0.0, 0.0, 0.0, 0.0, 0.0, 0.0, 0.0, 0.0, 0.0, 0.0, 0.0, 0.0, 0.0, 0.0, 0.0, 0.0, 0.0, 0.0, 0.0, 0.0, 0.0, 0.0, 0.0, 0.0, 0.0, 0.0, 0.0, 0.0, 0.0, 0.0, 0.0, 0.0, 0.0, 0.0, 0.0, 0.0, 0.0, 0.0, 0.0, 0.0, 0.0, 0.0, 0.0, 0.0, 0.0, 0.0, 0.0, 0.0, 0.0, 0.0, 0.0, 0.0, 0.0, 0.0, 0.0, 0.0, 0.0, 0.0, 0.0, 0.0, 0.0, 0.0, 0.0, 0.0, 0.0, 0.0, 0.0, 0.0, 0.0, 0.0, 0.0, 0.0, 0.0, 0.0, 0.0, 0.0, 0.0, 0.0, 0.0, 0.0, 0.0, 0.0, 0.0, 0.0, 0.0, 0.0, 0.0, 0.0, 0.0, 0.0, 0.0, 0.0, 0.0, 0.0, 0.0, 0.0, 0.0, 0.0, 0.0, 0.0, 0.0, 0.0, 0.0, 0.0, 0.0, 0.0, 0.0, 0.0, 0.0, 0.0, 0.0, 0.0, 0.0, 0.0, 0.0, 0.0, 0.0, 0.0, 0.0, 0.0, 0.0, 0.0, 0.0, 0.0, 0.0, 0.0, 0.0, 0.0, 0.0, 0.0, 0.0, 0.0, 0.0, 0.0, 0.0, 0.0, 0.0, 0.0, 0.0, 0.0, 0.0, 0.0, 0.0, 0.0, 0.0, 0.0, 0.0, 0.0, 0.0, 0.0, 0.0, 0.0, 0.0, 0.0, 0.0, 0.0, 0.0, 0.0, 0.0, 0.0, 0.0, 0.0, 0.0, 0.0, 0.0, 0.0, 0.0, 0.0, 0.0, 0.0, 0.0, 0.0, 0.0, 0.0, 0.0, 0.0, 0.0, 0.0, 0.0, 0.0, 0.0, 0.0, 0.0, 0.0, 0.0, 0.0, 0.0, 0.0, 0.0, 0.0, 0.0, 0.0, 0.0, 0.0, 0.0, 0.0, 0.0, 0.0, 0.0, 0.0, 0.0, 0.0, 0.0, 0.0, 0.0, 0.0, 0.0, 0.0, 0.0, 0.0, 0.0, 0.0, 0.0, 0.0, 0.0, 0.0, 0.0, 0.0, 0.0, 0.0, 0.0, 0.0, 0.0, 0.0, 0.0, 0.0, 0.0, 0.0, 0.0, 0.0, 0.0, 0.0, 0.0, 0.0, 0.0, 0.0, 0.0, 0.0, 0.0, 0.0, 0.0, 0.0, 0.0, 0.0, 0.0, 0.0, 0.0, 0.0, 0.0, 0.0, 0.0, 0.0, 0.0, 0.0, 0.0, 0.0, 0.0, 0.0, 0.0, 0.0, 0.0, 0.0, 0.0, 0.0, 0.0, 0.0, 0.0, 0.0, 0.0, 0.0, 0.0, 0.0, 0.0, 0.0, 0.0, 0.0, 0.0, 0.0, 0.0, 0.0, 0.0, 0.0, 0.0, 0.0, 0.0, 0.0, 0.0, 0.0, 0.0, 0.0, 0.0, 0.0, 0.0, 0.0, 0.0, 0.0, 0.0, 0.0, 0.0, 0.0, 0.0, 0.0, 0.0, 0.0, 0.0, 0.0, 0.0, 0.0, 0.0, 0.0, 0.0, 0.0, 0.0, 0.0, 0.0, 0.0, 0.0, 0.0, 0.0, 0.0, 0.0, 0.0, 0.0, 0.0, 0.0, 0.0, 0.0, 0.0, 0.0, 0.0, 0.0, 0.0, 0.0, 0.0, 0.0, 0.0, 0.0, 0.0, 0.0, 0.0, 0.0, 0.0, 0.0, 0.0, 0.0, 0.0, 0.0, 0.0, 0.0, 0.0, 0.0, 0.0, 0.0, 0.0, 0.0, 0.0, 0.0, 0.0, 0.0, 0.0, 0.0, 0.0, 0.0, 0.0, 0.0, 0.0, 0.0, 0.0, 0.0, 0.0, 0.0, 0.0, 0.0, 0.0, 0.0, 0.0, 0.0, 0.0, 0.0, 0.0, 0.0, 0.0, 0.0, 0.0, 0.0, 0.0, 0.0, 0.0, 0.0, 0.0, 0.0, 0.0, 0.0, 0.0, 0.0, 0.0, 0.0, 0.0, 0.0, 0.0, 0.0, 0.0, 0.0, 0.0, 0.0, 0.0, 0.0, 0.0, 0.0, 0.0, 0.0, 0.0, 0.0, 0.0, 0.0, 0.0, 0.0, 0.0, 0.0, 0.0, 0.0, 0.0, 0.0, 0.0, 0.0, 0.0, 0.0, 0.0, 0.0, 0.0, 0.0, 0.0, 0.0, 0.0, 0.0, 0.0, 0.0, 0.0, 0.0, 0.0, 0.0, 0.0, 0.0, 0.0, 0.0, 0.0, 0.0, 0.0, 0.0, 0.0, 0.0, 0.0, 0.0, 0.0, 0.0, 0.0, 0.0, 0.0, 0.0, 0.0, 0.0, 0.0, 0.0, 0.0, 0.0, 0.0, 0.0, 0.0, 0.0, 0.0, 0.0, 0.0, 0.0, 0.0, 0.0, 0.0, 0.0, 0.0, 0.0, 0.0, 0.0, 0.0, 0.0, 0.0, 0.0], "InitializationProduction"=[0.0, 0.0, 0.0, 0.0, 0.0, 0.0, 0.0, 0.0, 0.0, 0.0, 0.0, 0.0, 0.0, 0.0, 0.0, 0.0, 0.0, 0.0, 0.0, 0.0, 0.0]}  # InitializationValue-PieCahrt
            w363 = T15 {"InitializationDefect"=[0.0, 0.0, 0.0, 0.0, 0.0, 0.0, 0.0, 0.0, 0.0, 0.0, 0.0, 0.0, 0.0, 0.0, 0.0, 0.0, 0.0, 0.0, 0.0, 0.0, 0.0, 0.0, 0.0, 0.0, 0.0, 0.0, 0.0, 0.0, 0.0, 0.0, 0.0, 0.0, 0.0, 0.0, 0.0, 0.0, 0.0, 0.0, 0.0, 0.0, 0.0, 0.0, 0.0, 0.0, 0.0, 0.0, 0.0, 0.0, 0.0, 0.0, 0.0, 0.0, 0.0, 0.0, 0.0, 0.0, 0.0, 0.0, 0.0, 0.0, 0.0, 0.0, 0.0, 0.0, 0.0, 0.0, 0.0, 0.0, 0.0, 0.0, 0.0, 0.0, 0.0, 0.0, 0.0, 0.0, 0.0, 0.0, 0.0, 0.0, 0.0, 0.0, 0.0, 0.0, 0.0, 0.0, 0.0, 0.0, 0.0, 0.0, 0.0, 0.0, 0.0, 0.0, 0.0, 0.0, 0.0, 0.0, 0.0, 0.0, 0.0, 0.0, 0.0, 0.0, 0.0, 0.0, 0.0, 0.0, 0.0, 0.0, 0.0, 0.0, 0.0, 0.0, 0.0, 0.0, 0.0, 0.0, 0.0, 0.0, 0.0, 0.0, 0.0, 0.0, 0.0, 0.0, 0.0, 0.0, 0.0, 0.0, 0.0, 0.0, 0.0, 0.0, 0.0, 0.0, 0.0, 0.0, 0.0, 0.0, 0.0, 0.0, 0.0, 0.0, 0.0, 0.0, 0.0, 0.0, 0.0, 0.0, 0.0, 0.0, 0.0, 0.0, 0.0, 0.0, 0.0, 0.0, 0.0, 0.0, 0.0, 0.0, 0.0, 0.0, 0.0, 0.0, 0.0, 0.0, 0.0, 0.0, 0.0, 0.0, 0.0, 0.0, 0.0, 0.0, 0.0, 0.0, 0.0, 0.0, 0.0, 0.0, 0.0, 0.0, 0.0, 0.0, 0.0, 0.0, 0.0, 0.0, 0.0, 0.0, 0.0, 0.0, 0.0, 0.0, 0.0, 0.0, 0.0, 0.0, 0.0, 0.0, 0.0, 0.0, 0.0, 0.0, 0.0, 0.0, 0.0, 0.0, 0.0, 0.0, 0.0, 0.0, 0.0, 0.0, 0.0, 0.0, 0.0, 0.0, 0.0, 0.0, 0.0, 0.0, 0.0, 0.0, 0.0, 0.0, 0.0, 0.0, 0.0, 0.0, 0.0, 0.0, 0.0, 0.0, 0.0, 0.0, 0.0, 0.0, 0.0, 0.0, 0.0, 0.0, 0.0, 0.0, 0.0, 0.0, 0.0, 0.0, 0.0, 0.0, 0.0, 0.0, 0.0, 0.0, 0.0, 0.0, 0.0, 0.0, 0.0, 0.0, 0.0, 0.0, 0.0, 0.0, 0.0, 0.0, 0.0, 0.0, 0.0, 0.0, 0.0, 0.0, 0.0, 0.0, 0.0, 0.0, 0.0, 0.0, 0.0, 0.0, 0.0, 0.0, 0.0, 0.0, 0.0, 0.0, 0.0, 0.0, 0.0, 0.0, 0.0, 0.0, 0.0, 0.0, 0.0, 0.0, 0.0, 0.0, 0.0, 0.0, 0.0, 0.0, 0.0, 0.0, 0.0, 0.0, 0.0, 0.0, 0.0, 0.0, 0.0, 0.0, 0.0, 0.0, 0.0, 0.0, 0.0, 0.0, 0.0, 0.0, 0.0, 0.0, 0.0, 0.0, 0.0, 0.0, 0.0, 0.0, 0.0, 0.0, 0.0, 0.0, 0.0, 0.0, 0.0, 0.0, 0.0, 0.0, 0.0, 0.0, 0.0, 0.0, 0.0, 0.0, 0.0, 0.0, 0.0, 0.0, 0.0, 0.0, 0.0, 0.0, 0.0, 0.0, 0.0, 0.0, 0.0, 0.0, 0.0, 0.0, 0.0, 0.0, 0.0, 0.0, 0.0, 0.0, 0.0, 0.0, 0.0, 0.0, 0.0, 0.0, 0.0, 0.0, 0.0, 0.0, 0.0, 0.0, 0.0, 0.0, 0.0, 0.0, 0.0, 0.0, 0.0, 0.0, 0.0, 0.0, 0.0, 0.0, 0.0, 0.0, 0.0, 0.0, 0.0, 0.0, 0.0, 0.0, 0.0, 0.0, 0.0, 0.0, 0.0, 0.0, 0.0, 0.0, 0.0, 0.0, 0.0, 0.0, 0.0, 0.0, 0.0, 0.0, 0.0, 0.0, 0.0, 0.0, 0.0, 0.0, 0.0, 0.0, 0.0, 0.0, 0.0, 0.0, 0.0, 0.0, 0.0, 0.0, 0.0, 0.0, 0.0, 0.0, 0.0, 0.0, 0.0, 0.0, 0.0, 0.0, 0.0, 0.0, 0.0, 0.0, 0.0, 0.0, 0.0, 0.0, 0.0, 0.0, 0.0, 0.0, 0.0, 0.0, 0.0, 0.0, 0.0, 0.0, 0.0, 0.0, 0.0, 0.0, 0.0, 0.0, 0.0, 0.0, 0.0, 0.0, 0.0, 0.0, 0.0, 0.0, 0.0, 0.0, 0.0, 0.0, 0.0, 0.0, 0.0, 0.0, 0.0, 0.0, 0.0, 0.0, 0.0, 0.0, 0.0, 0.0, 0.0, 0.0, 0.0, 0.0, 0.0, 0.0, 0.0, 0.0, 0.0, 0.0, 0.0], "InitializationProduction"=[0.0, 0.0, 0.0, 0.0, 0.0, 0.0, 0.0, 0.0, 0.0, 0.0, 0.0, 0.0, 0.0, 0.0, 0.0, 0.0, 0.0, 0.0, 0.0, 0.0, 0.0]}  # InitializationValue-Barplot
            # "Triggered with Stop Button Press"
            n99 = call "Json_Specific part.vi"("error in (no error)"=w376, "Zen Analytics in"=w366, "JSON Cluster"=w371, "Part-num"=w378) -> ("error out"=w375:errorcluster, "Json Part no specicific op"=w377:T21)  [unwired: 6 in]
            n100 = Unbundle By Name(w377) -> ("Array Params.RowsIn2DArray"=w380:i32, "Array Params.SamplesToDisplay"=w368:i32, "Array Params.ColumnsIn2DArray"=w360:i32, "Array Params.UpdateRate"=w382:string, "PlotParameters"=w367:T19)
            n101 = call "String To Enum.vi"("error in (no error)"=w375, "string"=w382) -> ("error out"=w370:errorcluster, "Select Update Rate"=w372:enum16{"HIGH", "MEDIUM", "LOW"})  [unwired: 8 in]
            n102 = Decrement(x=w360) -> (x-1=w359:i32)
            n103 = Initialize Array(nan ("element"), w380, w360) -> (w379:dbl[][])
            n104 = call "Rate to Sampls&Time.vi"("error in (no error)"=w370, "JSON Cluster"=w371, "Select Update Rate"=w372) -> ("error out"=w369:errorcluster, "TimeElapsed"=w373:i32, "SampleElapsed"=w374:i32)  [unwired: 6 in]
            n105 = Divide(x=w359, y=2) -> (x/y=w358:dbl)
            n106 = Initialize Array(T7 {"SumOfSquareOfData"=0.0, "SumOfMeasurementData"=0.0, "N "=0} ("Cluster"), w358) -> (w357:T13)
          }
        }
        n107 = call "AnalyticsParamCluster.vi"("error in (no error)"=w295, "Number of columns"=w277, "MeasurementData"=w278) -> ("error out"=w286:errorcluster, "Initialization Data"=w285:T14, "x-y"=w308:i32)  [unwired: 6 in]
        n108 = call <vilib>:"Add State(s) to Queue__JKI_lib_State_Machine.vi"("State(s) in (\"\")"=w310) -> ("States Out"=w309:string)  [unwired: 14 in]
        n109 = case shown="True" w300 {
          tunnel: w277 -> [_ w328]
          tunnel: w285 -> [_ w326]
          tunnel: w308 -> [_ w324]
          tunnel: [w318 w322] -> w284
          tunnel: w297 -> [w318 _]
          tunnel: w286 -> [w317 w320]
          tunnel: [w317 w319] -> w281
          frame False {
          }
          frame True {
            n110 = Unbundle By Name(w326) -> ("Measurement-ID"=w325:i32[])
            n111 = Divide(x=w328, y=2) -> (x/y=w329:dbl)
            n112 = Increment(x=w329) -> (x+1=w321:dbl)
            n113 = Initialize Array(0.0 ("element"), w321) -> (w323:dbl[])
            n114 = call "DataArrangement(ID).vi"("error in (no error)"=w320, "y"=w324, "ID"=w325, "InputData"=w323) -> ("error out"=w319:errorcluster, "OutputData"=w322:dbl[])  [unwired: 6 in]
          }
        }
        n115 = Bundle By Name(cluster=w279, "InitializationParams.ColumnNo"=w277, "InitializationParams.MeasurementData"=w278) -> (w276:T1)
        n116 = Bundle By Name(cluster=w294, "InitializationValue-PieCahrt"=w270, "InitializationValue-Barplot"=w269, "Plot Cluster.ResultData2D"=w274, "clusterForShiftReg.Read Config"=FALSE ("Read Config"), "clusterForShiftReg.Re-initialized"=w316, "clusterForShiftReg.Plot:Present Terminal"=w315, "clusterForShiftReg.Prev Terminal Count"=w272, "clusterForShiftReg.Initialize 2D Array"=w274, "clusterForShiftReg.Timeout?"=w311, "clusterForShiftReg.Analytics Button Pressed?"=w312, "clusterForShiftReg.Analytics Or Back?"=w313, "JSON Cluster.Rows In 2D Array"=w293, "JSON Cluster.Samples To Display"=w292, "JSON Cluster.Columns In 2D Array"=w277, "JSON Cluster.Update Rate (Samples)"=w291, "JSON Cluster.Update Rate (Time)"=w290, "JSON Cluster.PlotParameters"=w289, "JSON Cluster.CurrentPartNumber"=w288, "JSON Cluster.MeasurementData"=w278, "Data & ID's"=w285, "InitializationValue-PieCahrt.InitializationDefect"=w284, "InitializationValue-PieCahrt.InitializationDefect"=w284, "StatDataIn"=w264, "StatData Old"=w264) -> (w283:T12)
        n117 = Generate User Event(user event=w275, event data cluster=w276, error in=w281) -> (error out=w280:errorcluster)  [unwired: 1 in, 1 out]
      }
      frame "ZenAnalytics : GraphRefference" {
        w395 = T5 {"HistgramGraph-reff"=[], "BarGraph-reff"=[], "PieGraph-reff"=[], "Lable-reff"=[], "TrendGraph-reff"=[], "CpCpkTable"=refnum}  # GraphRefference
        # "Getting grapg refference from UI panel"
        n118 = Unbundle By Name(w397) -> ("InterActorData"=w398:variant)
        n119 = Variant To Data(error in=w400, type=w395, Variant=w398) -> (data=w394:T5, error out=w399:errorcluster)
        n120 = Concatenate Strings("Graph reference not available\nCheck JSON file path/File name !" ("SolutionForError"), "\r", "ErrorCode:", "0X0E00A103" ("ErrorCode")) -> (w387:string)
        n121 = Bundle By Name(cluster=w397, "GraphRefference"=w394) -> (w396:T12)
        n122 = Bundle By Name(cluster=T4 {"Actor Info"={"Analytics Enqueuer"=refnum, "This VI"=refnum, "Module name"=""}, "Statistical Info"=[], "Graph Refference's"={"HistgramGraph-reff"=[], "BarGraph-reff"=[], "PieGraph-reff"=[], "Lable-reff"=[], "TrendGraph-reff"=[], "CpCpkTable"=refnum}, "ErrorMessage"=""} ("Analytics Information"), "ErrorMessage"=w387) -> (w386:T4)
        n123 = call-poly <userlib>:"Empty Array__ogtk.vi"("Array"=w394) -> ("Empty Array?"=w393:bool)  [unwired: 8 in]
        n124 = call <vilib>:"Add State(s) to Queue__JKI_lib_State_Machine.vi"("State(s) in (\"\")"=w401) -> ("States Out"=w402:string)  [unwired: 14 in]
        n125 = case shown="True" w393 {
          tunnel: w392 -> [_ w405]
          tunnel: w386 -> [_ w404]
          tunnel: "ERROR_INFO" ("State") -> [_ w403]
          frame False {
          }
          frame True {
            n126 = call "Output_ZA.vi"("State"=w403, "Analytics Information"=w404, "Zen Analytics in"=w405) -> ()  [unwired: 7 in, 2 out]
          }
        }
      }
      frame "ZenAnalytics : MeasurementName" {
        # "Checking user selected measurement name and taking the index of it"
        n127 = Unbundle By Name(w413) -> ("Data & ID's.Measurement Names"=w407:string[], "InterActorData"=w414:variant)
        n128 = Variant To Data(error in=w416, type="", Variant=w414) -> (data=w409:string, error out=w415:errorcluster)
        n129 = Search 1D Array(1D array=w407, element=w409, start index (0)=0) -> (index of element=w408:i32)
        n130 = Bundle By Name(cluster=w413, "IndexOfMeasurement"=w408) -> (w412:T12)
        n131 = call <vilib>:"Add State(s) to Queue__JKI_lib_State_Machine.vi"("State(s) in Front (\"\")"="ZenAnalytics : GetData" ("State(s) in Front (\"\")"), "State(s) in (\"\")"=w417) -> ("States Out"=w418:string)  [unwired: 13 in]
      }
      frame "ZenAnalytics : ResultData" {
        # "Getting the inspection result data from parent actor"
        n132 = Unbundle By Name(w423) -> ("ResultCluster"=w420:T16, "InterActorData"=w424:variant)
        n133 = Variant To Data(error in=w426, type=w420, Variant=w424) -> (data=w419:T16, error out=w425:errorcluster)
        n134 = Bundle By Name(cluster=w423, "ResultCluster"=w419) -> (w422:T12)
        n135 = call <vilib>:"Add State(s) to Queue__JKI_lib_State_Machine.vi"("State(s) in Front (\"\")"="ZenAnalytics : GetData" ("State(s) in Front (\"\")"), "State(s) in (\"\")"=w427) -> ("States Out"=w428:string)  [unwired: 13 in]
      }
      frame "ZenAnalytics : GetData" {
        # "Generating ID's and updating result in circular buffer and in case of analytics button is true then passing result data to plot.vi"
        n136 = Unbundle By Name(w472) -> ("oldTerminalCount"=w434:i32, "clusterForShiftReg.Initialize 2D Array"=w438:dbl[][], "clusterForShiftReg.Analytics Button Pressed?"=w471:bool, "clusterForShiftReg.Re-initialized"=w470:bool, "clusterForShiftReg.Prev Terminal Count"=w469:u32, "clusterForShiftReg.Plot:Present Terminal"=w468:u32, "JSON Cluster.Samples To Display"=w467:i32, "JSON Cluster.Rows In 2D Array"=w466:i32, "JSON Cluster.Update Rate (Time)"=w465:i32, "JSON Cluster.Update Rate (Samples)"=w437:i32, "JSON Cluster.PlotParameters"=w464:T19, "JSON Cluster.MeasurementData"=w463:T20, "Plot Cluster"=w451:T11, "ResultCluster.Terminal Count"=w433:u32, "ResultCluster.isPass"=w462:bool, "ResultCluster.Terminal Data 1D"=w461:dbl[], "ResultCluster.Defect"=w460:bool[], "Data & ID's"=w452:T14, "IndexOfMeasurement"=w453:i32, "GraphRefference"=w454:T5, "InitializationValues"=w455:dbl[][], "InitializationValue-PieCahrt"=w457:T15, "InitializationValue-Barplot"=w456:T15, "JSON Cluster.Columns In 2D Array"=w449:i32, "StatDataIn"=w430:T13, "StatData Old"=w431:T13)
        "Terminal Count" <- w433
        n137 = Unbundle By Name(w452) -> ("Measurement-ID"=w441:i32[])
        n138 = Equal?(x=w434, y=w433) -> (x = y?=w432:bool)
        n139 = call "Concatenate to 1D.vi"("Numberofcolumns"=w449, "ID"=w441, "error in (no error)"=w474, "Defect"=w460, "Terminal Data 1D"=w461, "isPass"=w462) -> ("error out"=w485:errorcluster, "1D Concatenated Array"=w436:dbl[])  [unwired: 4 in]
        n140 = call <vilib>:"Add State(s) to Queue__JKI_lib_State_Machine.vi"("State(s) in (\"\")"=w487) -> ("States Out"=w486:string)  [unwired: 14 in]
        n141 = Select(t=w431, s=w432, f=w430) -> (s? t:f=w429:T13)
        n142 = call "Replace and Reduce Array.vi"("dimension size"=w466, "initialized 2D in"=w438, "error in"=w485, "rows to display"=w467, "tc"=w433, "1D array"=w436) -> ("error out"=w482:errorcluster, "start index"=w484:u32, "reduced 2D"=w481:dbl[][], "initialized 2D out"=w447:dbl[][])  [unwired: 2 in]
        "Reduced 2D" <- w481
        n143 = call "Cumulative StatisticalParamets.vi"("N"=w433, "error in (no error)"=w482, "Measurement Data"=w436, "DataIn"=w429, "Initialization Data"=w452) -> ("error out"=w450:errorcluster, "DataOut"=w435:T13, "Statistical Parameters"=w443:string[][])  [unwired: 4 in]
        n144 = call "Samples Elapsed.vi"("error in (no error)"=w450, "SE"=w437, "TC"=w433, "Present Terminal"=w469) -> ("error out"=w477:errorcluster, "Samples Elapsed"=w478:bool)  [unwired: 6 in]
        n145 = And(x=w471, y=w478) -> (x .and. y?=w479:bool)
        n146 = case shown="True" w479 {
          tunnel: [w495 w518] -> w476
          tunnel: w481 -> [_ w503]
          tunnel: w484 -> [_ w504]
          tunnel: w464 -> [_ w530]
          tunnel: [w496 w527] -> w459
          tunnel: w467 -> [_ w528]
          tunnel: w433 -> [_ w500]
          tunnel: w469 -> [w496 w523]
          tunnel: w477 -> [w495 w524]
          tunnel: [w494 w523] -> w458
          tunnel: w468 -> [w494 _]
          tunnel: w471 -> [_ w522]
          tunnel: [FALSE w521] -> w475
          tunnel: w470 -> [_ w520]
          tunnel: w443 -> [_ w519]
          tunnel: w452 -> [_ w510]
          tunnel: w455 -> [w489 w509]
          tunnel: w457 -> [w490 w508]
          tunnel: w456 -> [w491 w507]
          tunnel: [w489 w516] -> w445
          tunnel: [w491 w515] -> w446
          tunnel: [w490 w505] -> w448
          tunnel: w454 -> [_ w513]
          tunnel: w463 -> [_ w512]
          tunnel: w453 -> [_ w511]
          tunnel: [w492 w506] -> w473
          tunnel: w451 -> [w492 _]
          tunnel: w438 -> [_ w502]
          tunnel: [w488 TRUE] -> w442
          tunnel: [w488 FALSE] -> w440
          tunnel: w439 -> [_ w497]
          frame False {
            w488 = FALSE
          }
          frame True {
            w514 = T11 {"Reduced 2D"=[], "Start Index"=0, "No Of New Termnals"=0, "Top/Bottom"=FALSE, "Values Inserted"=0, "Re-Initialised"=FALSE, "Statistical params"=[], "MeasurementInitializationData"={"Measurement-ID"=[], "Measurement Names"=[], "NominalValues"=[], "LSL"=[], "USL"=[], "LCL"=[], "UCL"=[]}, "MeasurementData"=[], "ResultData2D"=[], "PlotParameters"={"Trend"=[], "Histogram"=[], "BarPlot"=[], "PieChart"=[]}}  # Plot Cluster
            w521 = TRUE  # Reset
            n147 = call "New Terminals Updated_1.vi"("Prev Terminal Count"=w523, "error in (no error)"=w524, "Analytics Button Pressed?"=w522, "Samples to display"=w528, "Terminal Count"=w500) -> ("error out"=w517:errorcluster, "Top/Bottom"=w525:bool, "Values Inserted"=w526:u32, "No Of New Terminals"=w529:u32, "Prev Terminal Count"=w527:u32)  [unwired: 2 in]
            n148 = Array Subset(array=w502, length (row)=w500) -> (w501:dbl[][])  [unwired: 3 in]
            n149 = Bundle By Name(cluster=w514, "ResultData2D"=w501, "Re-Initialised"=w520, "Reduced 2D"=w503, "Start Index"=w504, "PlotParameters"=w530, "MeasurementData"=w512, "No Of New Termnals"=w529, "Values Inserted"=w526, "Top/Bottom"=w525, "Statistical params"=w519, "MeasurementInitializationData"=w510) -> (w506:T11)
            n150 = call "Plot.vi"("Zen Analytics in"=w497, "IndexOfMeasurement"=w511, "InitializationValue-Input-Barplot"=w507, "InitializationValue-Input-PieCahrt"=w508, "error Input"=w517, "Initialization input"=w509, "Graph Refference's"=w513, "Plot Cluster"=w506) -> ("error output"=w518:errorcluster, "InitializationOutput"=w516:dbl[][], "InitializationValue-output-Barplot"=w515:T15, "InitializationValue-output-PieCahrt"=w505:T15)
          }
        }
        n151 = call "Time Elapsed.vi"("error in (no error)"=w476, "TE"=w465, "Reset"=w475) -> ("error out"=w480:errorcluster, "Timeout"=w444:bool)  [unwired: 7 in]
        n152 = Bundle By Name(cluster=w472, "oldTerminalCount"=w433, "Statistical Parameters"=w443, "clusterForShiftReg.Analytics Button Pressed?"=w442, "clusterForShiftReg.Re-initialized"=w440, "clusterForShiftReg.Prev Terminal Count"=w459, "clusterForShiftReg.Plot:Present Terminal"=w458, "Plot Cluster"=w473, "InitializationValues"=w445, "InitializationValue-Barplot"=w446, "clusterForShiftReg.Initialize 2D Array"=w447, "clusterForShiftReg.Timeout?"=w444, "InitializationValue-PieCahrt"=w448, "StatDataIn"=w435, "StatData Old"=w429) -> (w483:T12)
      }
      frame "ZenAnalytics : Analytics" {
        w534 = TRUE
        # "Analytics button event from parent actor and updating analytics UI"
        n153 = Unbundle By Name(w536) -> ("A_Count"=w543:i32, "clusterForShiftReg.Read Config"=w541:bool, "clusterForShiftReg.Initialize 2D Array"=w540:dbl[][], "clusterForShiftReg.Timeout?"=w539:bool, "clusterForShiftReg.Prev Terminal Count"=w538:u32, "clusterForShiftReg.Plot:Present Terminal"=w537:u32, "StatData Old"=w531:T13)
        n154 = Increment(x=w543) -> (x+1=w533:i32)
        n155 = Equal To 0?(x=w543) -> (x = 0?=w545:bool)
        n156 = case shown="False" w545 {
          tunnel: [FALSE TRUE] -> w544
          frame False {
          }
          frame True {
          }
        }
        n157 = Bundle By Name(cluster=w536, "clusterForShiftReg.Analytics Button Pressed?"=w534, "clusterForShiftReg.Analytics Or Back?"=w534, "clusterForShiftReg.Re-initialized"=w544, "clusterForShiftReg.Read Config"=w541, "clusterForShiftReg.Initialize 2D Array"=w540, "clusterForShiftReg.Timeout?"=w539, "clusterForShiftReg.Prev Terminal Count"=w538, "clusterForShiftReg.Plot:Present Terminal"=w537, "A_Count"=w533, "StatDataIn"=w531) -> (w535:T12)
        n158 = call <vilib>:"Add State(s) to Queue__JKI_lib_State_Machine.vi"("State(s) in Front (\"\")"="ZenAnalytics : GetData" ("State(s) in Front (\"\")"), "State(s) in (\"\")"=w547) -> ("States Out"=w546:string)  [unwired: 13 in]
      }
      frame "ZenAnalytics : Pause" {
        # "Analytics Paused"
        n159 = call <vilib>:"Add State(s) to Queue__JKI_lib_State_Machine.vi"("State(s) in (\"\")"=w553) -> ("States Out"=w552:string)  [unwired: 14 in]
      }
      frame "ZenAnalytics : StatisticalData" {
        # "Sending Statistical data to parent actor"
        n160 = Unbundle By Name(w565) -> ("Statistical Parameters"=w554:string[][], "InterActorData"=w559:variant)
        n161 = Variant To Data(error in=w558, type=TRUE ("StatisticalData"), Variant=w559) -> (data=w555:bool, error out=w557:errorcluster)
        n162 = Insert Into Array(array=w554, index (col)=0 ("disabled index (col)"), new element=string[] ["Mean", "Standard Deviation", "Variance", "Cp", "CpK"] ("new element/subarray")) -> (w562:string[][])  [unwired: 1 in]
        n163 = case shown="True" w555 {
          tunnel: w557 -> [w569 w576]
          tunnel: [w569 w575] -> w563
          tunnel: w566 -> [_ w572]
          tunnel: w562 -> [_ w573]
          frame False {
          }
          frame True {
            n164 = Bundle By Name(cluster=T4 {"Actor Info"={"Analytics Enqueuer"=refnum, "This VI"=refnum, "Module name"=""}, "Statistical Info"=[], "Graph Refference's"={"HistgramGraph-reff"=[], "BarGraph-reff"=[], "PieGraph-reff"=[], "Lable-reff"=[], "TrendGraph-reff"=[], "CpCpkTable"=refnum}, "ErrorMessage"=""} ("Analytics Information"), "Statistical Info"=w573) -> (w574:T4)
            n165 = call "Output_ZA.vi"("error in (no error)"=w576, "State"="STAT_INFO", "Analytics Information"=w574, "Zen Analytics in"=w572) -> ("error out"=w575:errorcluster)  [unwired: 6 in, 1 out]
          }
        }
        n166 = call <vilib>:"Add State(s) to Queue__JKI_lib_State_Machine.vi"("State(s) in (\"\")"=w568) -> ("States Out"=w567:string)  [unwired: 14 in]
        n167 = Bundle By Name(cluster=w565, "Statistical Parameters"=w554) -> (w564:T12)
      }
      frame "ZenAnalytics : GraphRefferenceForPrint" {
        # "Updatig charts and Sending Graphs refference data to parent actor"
        n168 = Unbundle By Name(w578) -> ("GraphRefference"=w582:T5)
        n169 = Bundle By Name(cluster=T4 {"Actor Info"={"Analytics Enqueuer"=refnum, "This VI"=refnum, "Module name"=""}, "Statistical Info"=[], "Graph Refference's"={"HistgramGraph-reff"=[], "BarGraph-reff"=[], "PieGraph-reff"=[], "Lable-reff"=[], "TrendGraph-reff"=[], "CpCpkTable"=refnum}, "ErrorMessage"=""} ("Analytics Information"), "Graph Refference's"=w582) -> (w581:T4)
        n170 = call "Output_ZA.vi"("error in (no error)"=w577, "State"="GRAPH_INFO", "Analytics Information"=w581, "Zen Analytics in"=w584) -> ("error out"=w583:errorcluster)  [unwired: 6 in, 1 out]
        n171 = call <vilib>:"Add State(s) to Queue__JKI_lib_State_Machine.vi"("State(s) in (\"\")"=w586) -> ("States Out"=w585:string)  [unwired: 14 in]
      }
      frame "ZenAnalytics : Back" {
        w587 = FALSE ("Analytics Or Back?")
        # "Stop updating the analytics UI"
        n172 = Unbundle By Name(w589) -> ("clusterForShiftReg.Re-initialized"=w595:bool, "clusterForShiftReg.Initialize 2D Array"=w594:dbl[][], "clusterForShiftReg.Timeout?"=w593:bool, "clusterForShiftReg.Read Config"=w592:bool, "clusterForShiftReg.Prev Terminal Count"=w591:u32, "clusterForShiftReg.Plot:Present Terminal"=w590:u32)  [unwired: 1 out]
        n173 = call <vilib>:"Add State(s) to Queue__JKI_lib_State_Machine.vi"("State(s) in (\"\")"=w597) -> ("States Out"=w596:string)  [unwired: 14 in]
        n174 = Bundle By Name(cluster=w589, "clusterForShiftReg.Analytics Or Back?"=w587, "clusterForShiftReg.Re-initialized"=w595, "clusterForShiftReg.Initialize 2D Array"=w594, "clusterForShiftReg.Timeout?"=w593, "clusterForShiftReg.Analytics Button Pressed?"=w587, "clusterForShiftReg.Read Config"=w592, "clusterForShiftReg.Prev Terminal Count"=w591, "clusterForShiftReg.Plot:Present Terminal"=w590) -> (w588:T12)
      }
      frame "ZenAnalytics : Stop" {
        w608 = u32 0 ("Prev Terminal Count")
        # "Stop analytics functionality"
        n175 = Unbundle By Name(w602) -> ("clusterForShiftReg.Re-initialized"=w606:bool, "clusterForShiftReg.Timeout?"=w605:bool, "clusterForShiftReg.Analytics Button Pressed?"=w604:bool, "clusterForShiftReg.Analytics Or Back?"=w603:bool)  [unwired: 1 out]
        n176 = call <vilib>:"Add State(s) to Queue__JKI_lib_State_Machine.vi"("State(s) in (\"\")"=w610) -> ("States Out"=w609:string)  [unwired: 14 in]
        n177 = Bundle By Name(cluster=w602, "clusterForShiftReg.Re-initialized"=w606, "clusterForShiftReg.Initialize 2D Array"=dbl[][] [], "clusterForShiftReg.Timeout?"=w605, "clusterForShiftReg.Analytics Button Pressed?"=w604, "clusterForShiftReg.Analytics Or Back?"=w603, "clusterForShiftReg.Read Config"=TRUE ("Read Config"), "clusterForShiftReg.Prev Terminal Count"=w608, "clusterForShiftReg.Plot:Present Terminal"=w608) -> (w601:T12)
      }
      frame "ZenAnalytics : Exit" {
        # "EXIT"
        n178 = call <vilib>:"Read Self Enqueuer.vi"("Actor"=w618) -> ("Self Enqueuer"=w617:refnum<class "Message Enqueuer.lvclass">)  [unwired: 10 in]
        n179 = Unregister For Events(event registration refnum=w614, error in=w613) -> (error out=w611:errorcluster)
        n180 = call <vilib>:"Send Normal Stop.vi"("error in (no error)"=w613, "Message Enqueuer"=w617) -> ("error out"=w616:errorcluster)  [unwired: 9 in]
        n181 = Merge Errors(w611, w616) -> (w612:errorcluster)
        n182 = call <vilib>:"Add State(s) to Queue__JKI_lib_State_Machine.vi"("State(s) in Front (\"\")"="Macro: Exit" ("State(s) in Front (\"\")"), "State(s) in (\"\")"=w620) -> ("States Out"=w621:string)  [unwired: 13 in]
      }
    }
  }
  n183 = call "UserInterface_ZA.vi"("error in"=w4, "Zen Analytics"="Zen Analytics in", "InitializationData"=w2) -> ("error out"=w10:errorcluster)  [unwired: 8 in]
  n184 = Merge Errors(w12, w1, w10) -> (→"error out":errorcluster)
